vi "Parameter.vi"(9 "In":string, 10 "VIId":string, 11 "VariablesRef":T3) -> ()   [LabVIEW 2018, in "File.lvlib"]
uses:
  File.lvlib
  <userlib>/_OpenG.lib/dictionary/dictionary.llb/Dictionary Object RefNum__ogtk.ctl
  <userlib>/_OpenG.lib/dictionary/dictionary.llb/Dictionary Object RefNum - Enum__ogtk.ctl
  <vilib>/addons/_JKI.lib/Serialization/JSON/JKI JSON Serialization.lvlib
panel:
  in  "Tab Control":enum32{"Config", "控件"}(tab)
  in  "Type":T1(tab)
  in  "路径类型_SetPath":u16(ring) items=["Relative", "Absolute"]
  in  "禁用缓存_CreatFile":bool
  in  "权限_CreatFile":u16(ring) caption="权限" items=["read/write", "read-only", "write-only"]
  in  "操作_CreatFile":u16(ring) caption="操作" items=["open", "replace", "create", "open or create", "replace or create", "replace or create with confirmation"]
  in  "手动确认_Delete":bool
  in  "完整层次结构_Delete":bool
  in  "计数_ReadTextFile":i32=-1 caption="计数"
  in  "文本_WriteTextFile":string(combo) caption="文本"
  in  "起始位置_WriteTextFile":u16(ring) caption="起始位置" items=["start", "end", "current"]
  in  "偏移_WriteTextFile":i64 caption="偏移"
  in  "计数_ReadBinFile":i32=-1 caption="计数"
  in  "字节顺序_ReadBinFile":u16(ring) caption="字节顺序" items=["big-endian, network order", "native, host order", "little-endian"]
  in  "前置数据大小_WriteBinFile":bool=TRUE
  in  "字节顺序_WriteBinFile":u16(ring) items=["big-endian, network order", "native, host order", "little-endian"]
  in  "二进制_WriteBinFile":string(combo) caption="二进制内容"
  in  "覆盖_Move":bool
  in  "文件路径_Move":string(combo) caption="目标文件路径"
  in  "目标文件路径_Copy":string(combo) caption="目标文件路径"
  in  "覆盖_Copy":bool
  in  "类型_ListFolder":u16(ring) caption="类型" items=["File", "Folder"]
  in  "方法(Method)":T2(ring)
  in  "路径(Path)":string(combo)
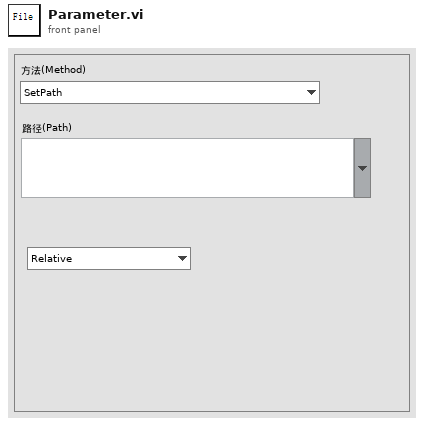
[diagram p1: front panel]
types:
  T1 = enum32{"SetPath", "CreatFile", "CreatFolder", "Delete", "ReadTextFile", "WriteTextFile", "ReadBinFile", "WriteBinFile", "ReadFileMD5", "Move", "Copy", "GetFileSize", "CheckifFileorFolderExists", "ListFolder"}
  T2 = enum16{"SetPath", "CreatFile", "CreatFolder", "Delete", "ReadTextFile", "WriteTextFile", "ReadBinFile", "WriteBinFile", "ReadFileMD5", "Move", "Copy", "GetFileSize", "CheckifFileorFolderExists", "ListFolder"}
  T3 = typedef "Dictionary Object RefNum__ogtk.ctl" = refnum<k1>
  T4 = cluster{"SetPath":cluster{"json":cluster{"Method":string, "Path":string, "PathType":string}}, "CreatFile":cluster{"json":cluster{"Method":string, "Path":string, "Operation":string, "Access":string, "DisableBuffering":bool}}, "CreatFolder":cluster{"json":cluster{"Method":string, "Path":string}}, "Delete":cluster{"json":cluster{"Method":string, "Path":string, "EntireHierarchy":bool, "Confirm":bool}}, "ReadTextFile":cluster{"json":cluster{"Method":string, "Path":string, "count":i32}}, "WriteTextFile":cluster{"json":cluster{"Method":string, "Path":string, "Offset":i64, "Position":string, "Text":string}}, "ReadBinFile":cluster{"json":cluster{"Method":string, "Path":string, "Count":i32, "ByteOrder":string}}, "WriteBinFile":cluster{"json":cluster{"Method":string, "Path":string, "ByteOrder":string, "PrependDataSize":bool, "Bin":string}}, "ReadFileMD5":cluster{"json":cluster{"Method":string, "Path":string}}, "Move":cluster{"json":cluster{"Method":string, "Path":string, "TargetPath":string, "Overwrite":bool}}, "Copy":cluster{"json":cluster{"Method":string, "Path":string, "TargetPath":string, "Overwrite":bool}}, "GetFileSize":cluster{"json":cluster{"Method":string, "Path":string}}, "CheckifFileorFolderExists":cluster{"json":cluster{"Method":string, "Path":string}}, "ListFolder":cluster{"json":cluster{"Method":string, "Path":string, "Type":string}}}
  T5 = enum32{"Invalid", "Standard", "Closed", "Hidden", "Minimized", "Maximized"}
  T6 = enum32{"invalid app kind", "Development System", "Run Time System", "Student Edition", "Embedded LabVIEW", "Evaluation", "Custom"}
  T7 = cluster{"Core":cluster{"Current VI Reference":refnum<vi>, "Close Panel on Exit?":bool}, "Parameter":cluster{"VariableRef":T3}, "Synchronize":cluster{"EnqueueData":cluster{"Action":enum16{"Create", "Query", "Revert", "UpdateVariable", "Close"}, "Data":variant}, "Echo":cluster{"VIRef":refnum<vi>, "JsonOut":string, "Status":string}, "Communicate":cluster{"ID":string, "JsonIn":string, "VarRef":T3}, "Queue":refnum<queue>}, "FileClusters":cluster{"SetPath":cluster{"json":cluster{"Method":string, "Path":string, "PathType":string}}, "CreatFile":cluster{"json":cluster{"Method":string, "Path":string, "Operation":string, "Access":string, "DisableBuffering":bool}}, "CreatFolder":cluster{"json":cluster{"Method":string, "Path":string}}, "Delete":cluster{"json":cluster{"Method":string, "Path":string, "EntireHierarchy":bool, "Confirm":bool}}, "ReadTextFile":cluster{"json":cluster{"Method":string, "Path":string, "count":i32}}, "WriteTextFile":cluster{"json":cluster{"Method":string, "Path":string, "Offset":i64, "Position":string, "Text":string}}, "ReadBinFile":cluster{"json":cluster{"Method":string, "Path":string, "Count":i32, "ByteOrder":string}}, "WriteBinFile":cluster{"json":cluster{"Method":string, "Path":string, "ByteOrder":string, "PrependDataSize":bool, "Bin":string}}, "ReadFileMD5":cluster{"json":cluster{"Method":string, "Path":string}}, "Move":cluster{"json":cluster{"Method":string, "Path":string, "TargetPath":string, "Overwrite":bool}}, "Copy":cluster{"json":cluster{"Method":string, "Path":string, "TargetPath":string, "Overwrite":bool}}, "GetFileSize":cluster{"json":cluster{"Method":string, "Path":string}}, "CheckifFileorFolderExists":cluster{"json":cluster{"Method":string, "Path":string}}, "ListFolder":cluster{"json":cluster{"Method":string, "Path":string, "Type":string}}}}
  T8 = cluster{"EnqueueData":cluster{"Action":enum16{"Create", "Query", "Revert", "UpdateVariable", "Close"}, "Data":variant}, "Echo":cluster{"VIRef":refnum<vi>, "JsonOut":string, "Status":string}, "Communicate":cluster{"ID":string, "JsonIn":string, "VarRef":T3}, "Queue":refnum<queue>}
  T9 = cluster{"Current VI Reference":refnum<vi>, "Close Panel on Exit?":bool}
  T10 = cluster{"json":cluster{"Method":string, "Path":string, "PathType":string}}
  T11 = cluster{"json":cluster{"Method":string, "Path":string, "Operation":string, "Access":string, "DisableBuffering":bool}}
  T12 = cluster{"json":cluster{"Method":string, "Path":string}}
  T13 = cluster{"json":cluster{"Method":string, "Path":string, "EntireHierarchy":bool, "Confirm":bool}}
  T14 = cluster{"json":cluster{"Method":string, "Path":string, "count":i32}}
  T15 = cluster{"json":cluster{"Method":string, "Path":string, "Offset":i64, "Position":string, "Text":string}}
  T16 = cluster{"json":cluster{"Method":string, "Path":string, "Count":i32, "ByteOrder":string}}
  T17 = cluster{"json":cluster{"Method":string, "Path":string, "ByteOrder":string, "PrependDataSize":bool, "Bin":string}}
  T18 = cluster{"json":cluster{"Method":string, "Path":string, "TargetPath":string, "Overwrite":bool}}
  T19 = cluster{"json":cluster{"Method":string, "Path":string, "Type":string}}
  T20 = cluster{"Action":enum16{"Create", "Query", "Revert", "UpdateVariable", "Close"}, "Data":variant}
  T21 = cluster{"ID":string, "JsonIn":string, "VarRef":T3}
  T22 = enum16{"Create", "Query", "Revert", "UpdateVariable", "Close"}
  T23 = cluster{"VIRef":refnum<vi>, "JsonOut":string, "Status":string}
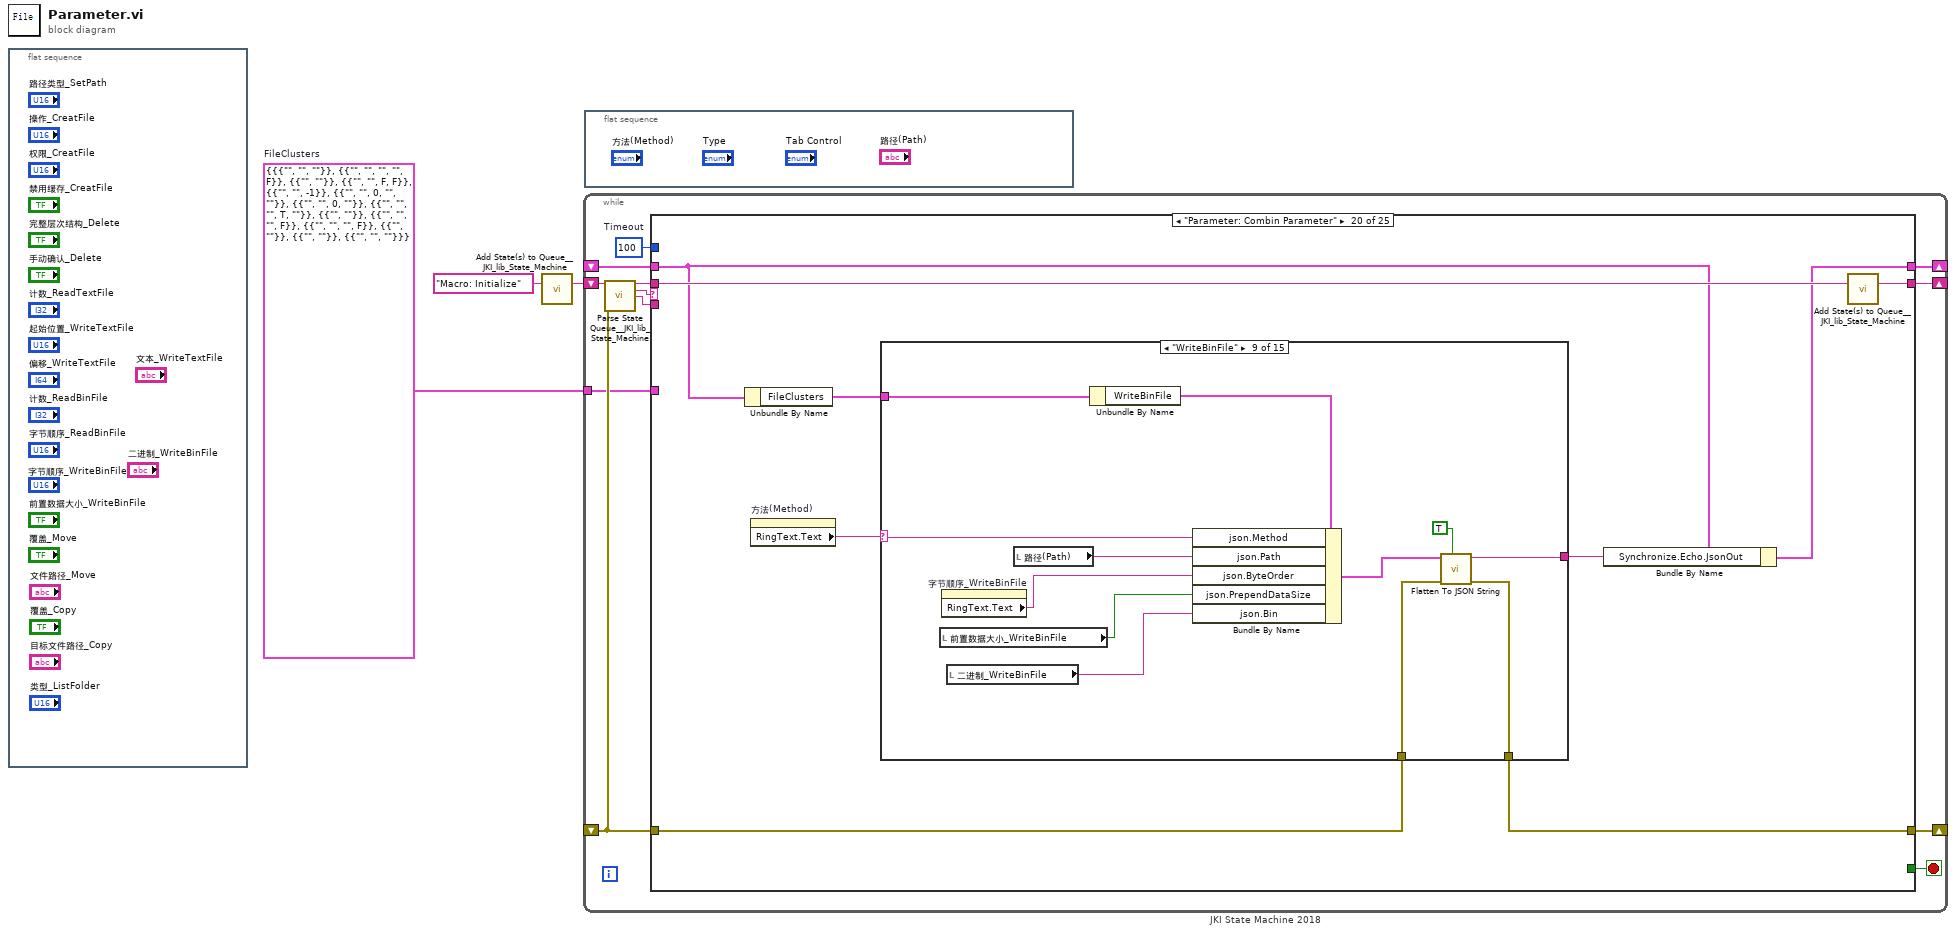
[diagram p0: block diagram]
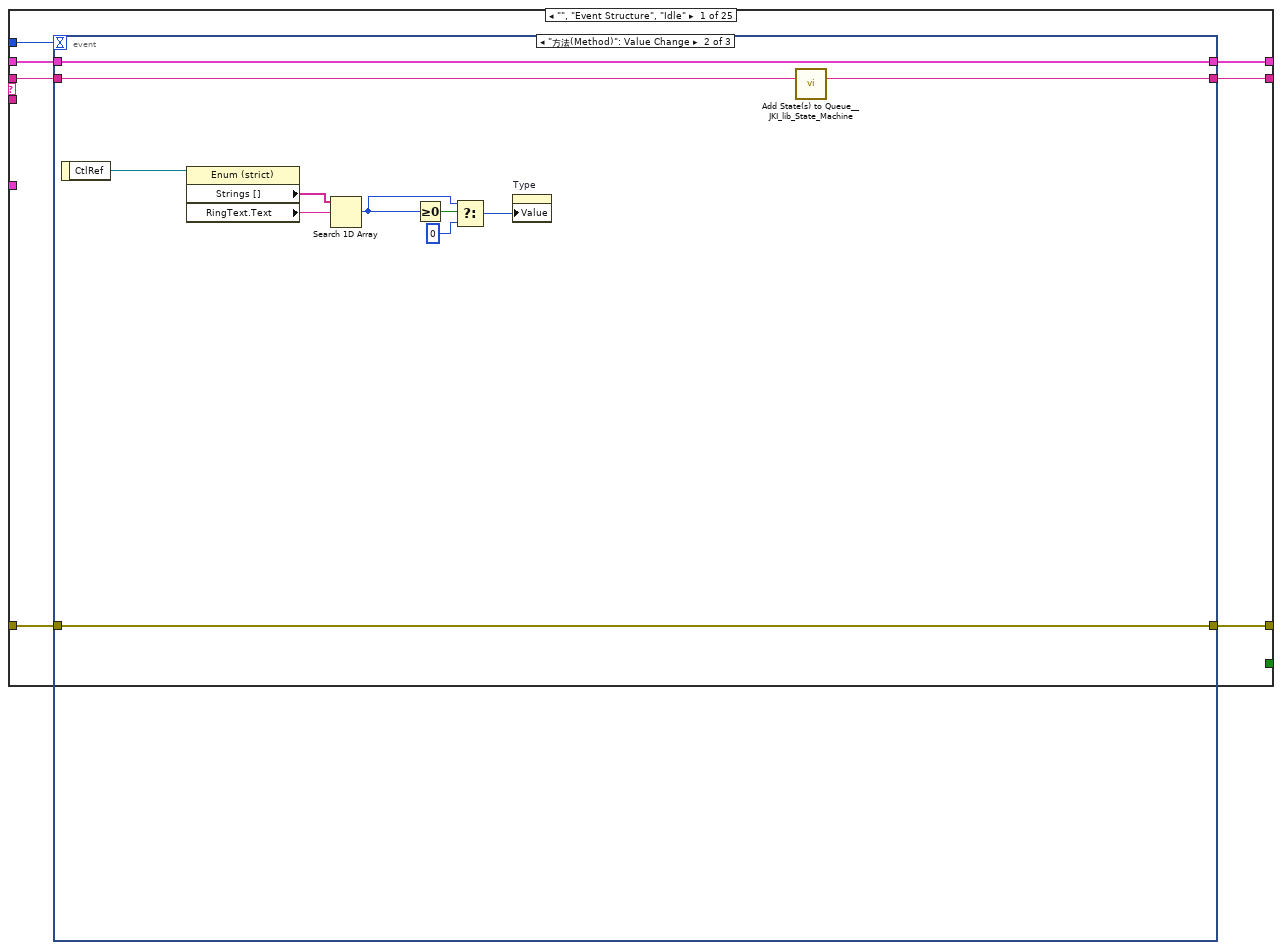
[diagram p2: hidden frame]
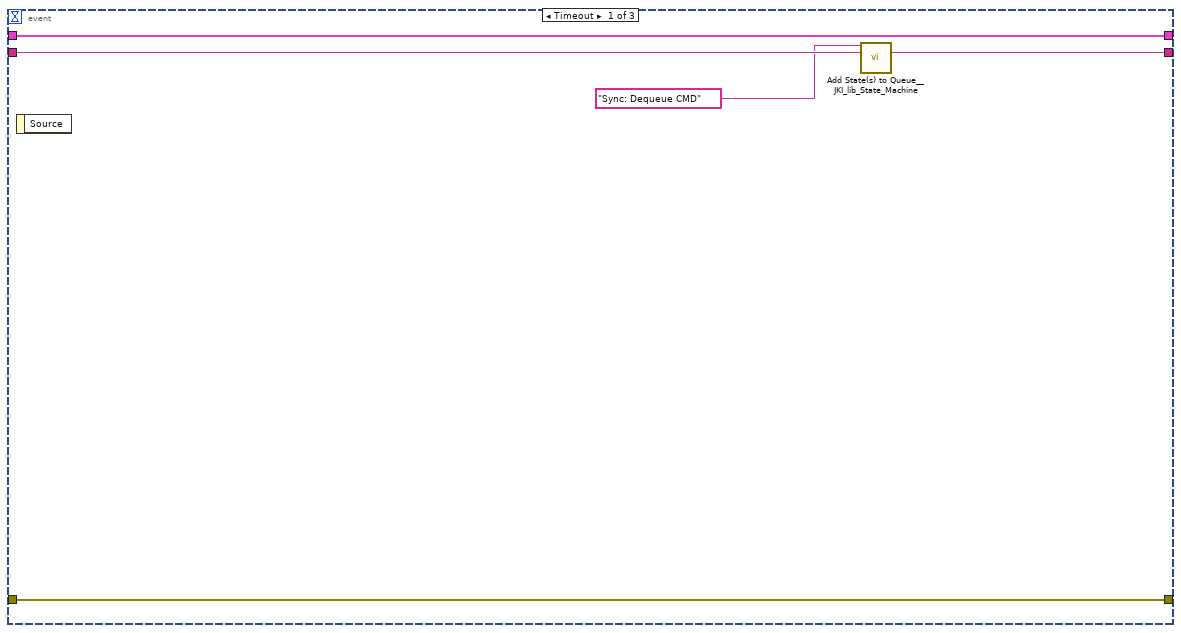
[diagram p3: hidden frame]
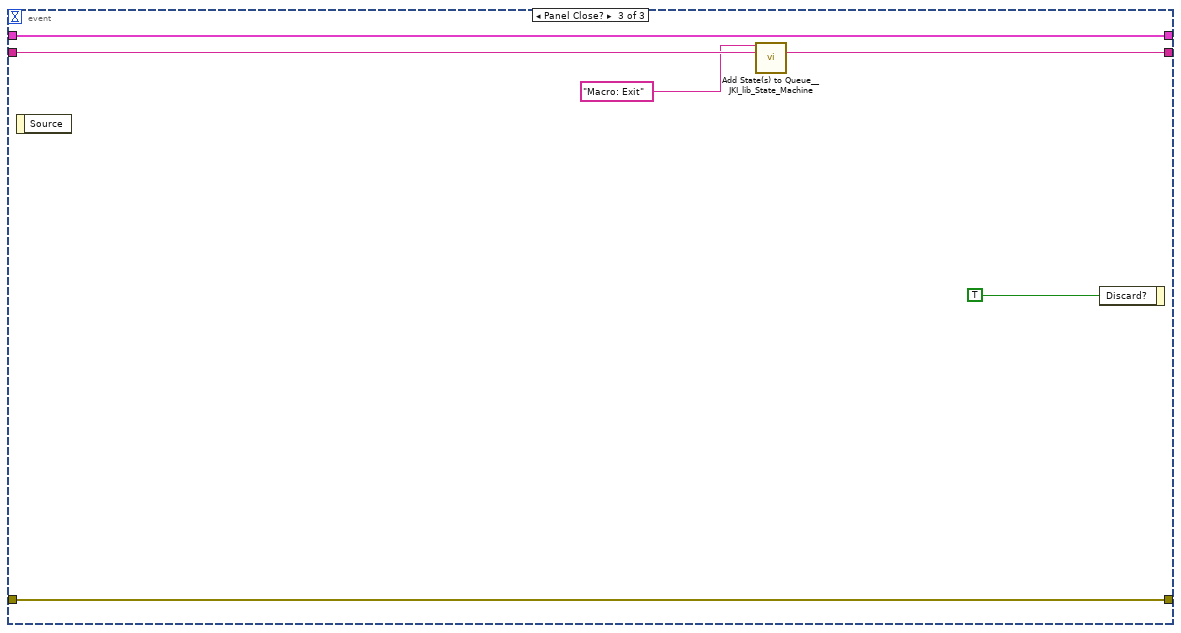
[diagram p4: hidden frame]
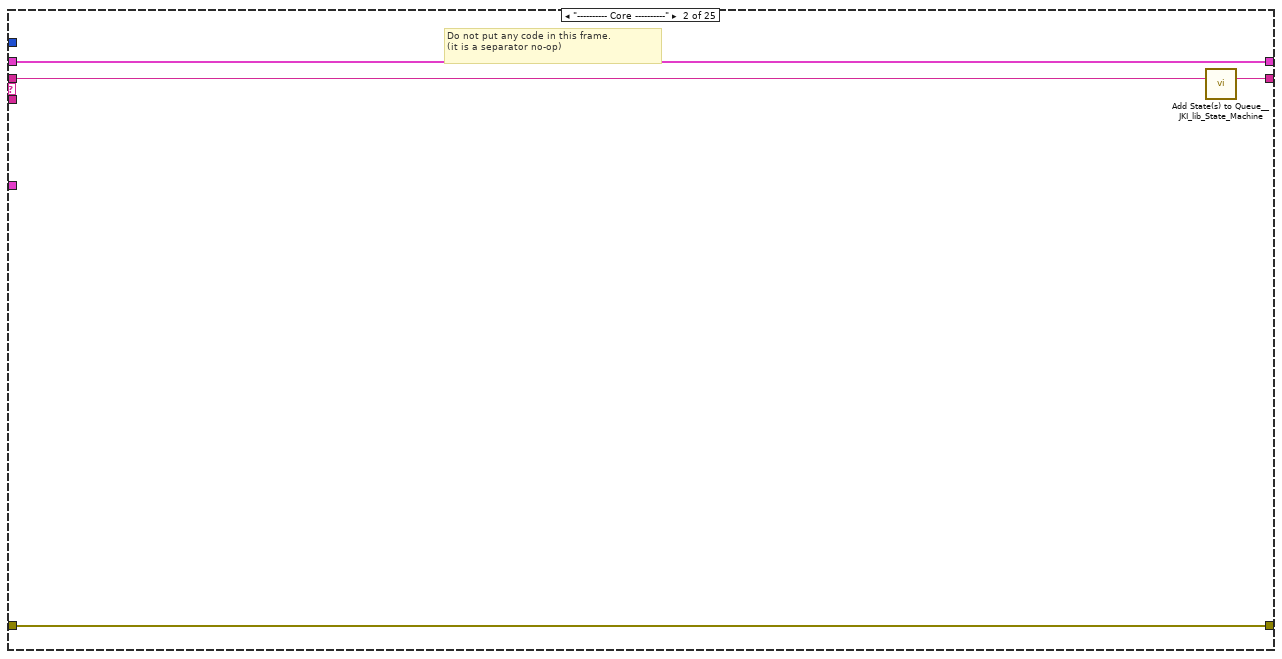
[diagram p5: hidden frame]
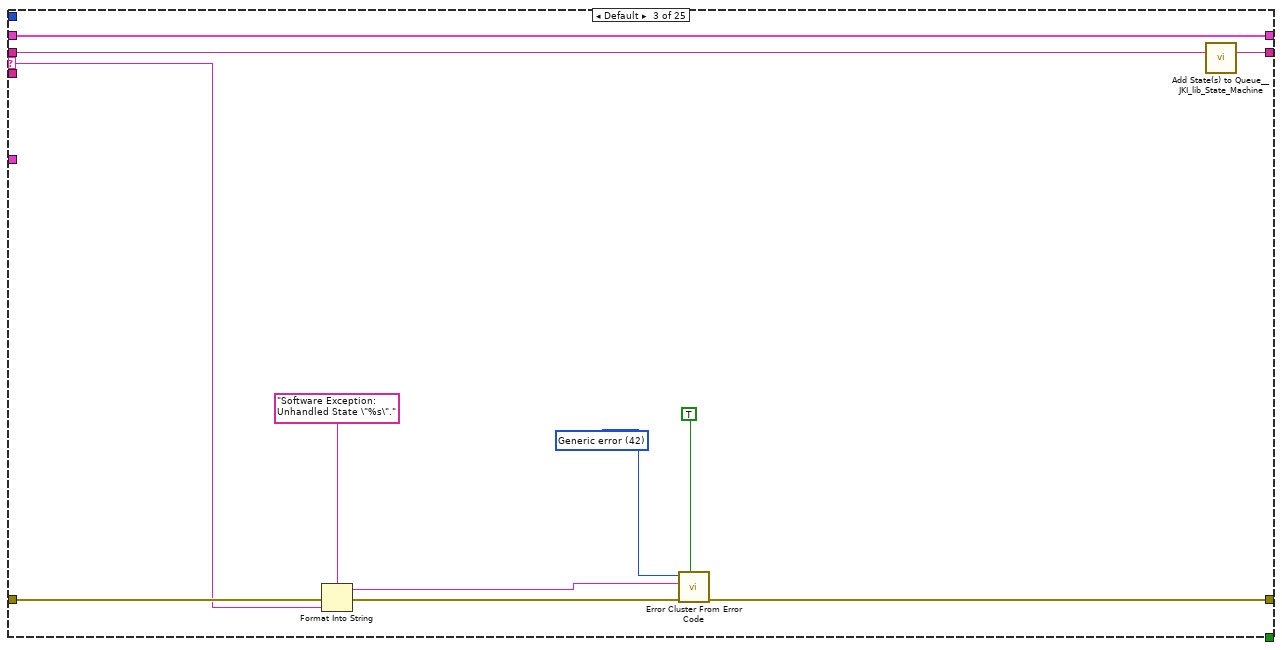
[diagram p6: hidden frame]
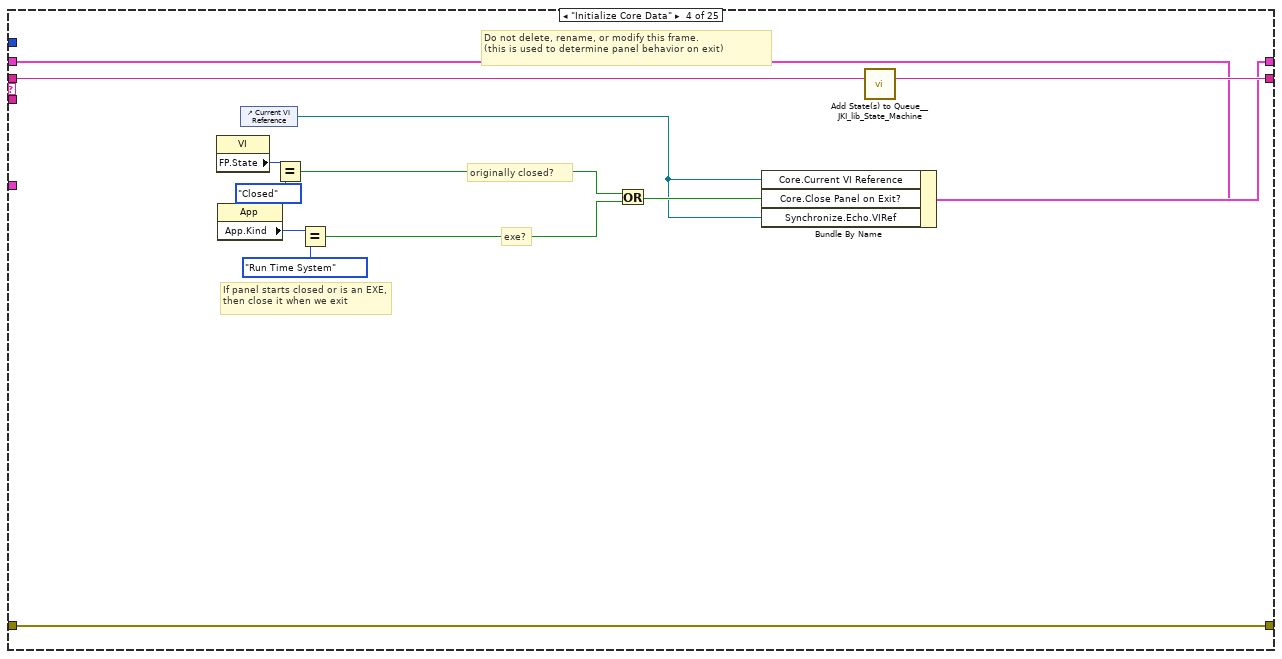
[diagram p7: hidden frame]
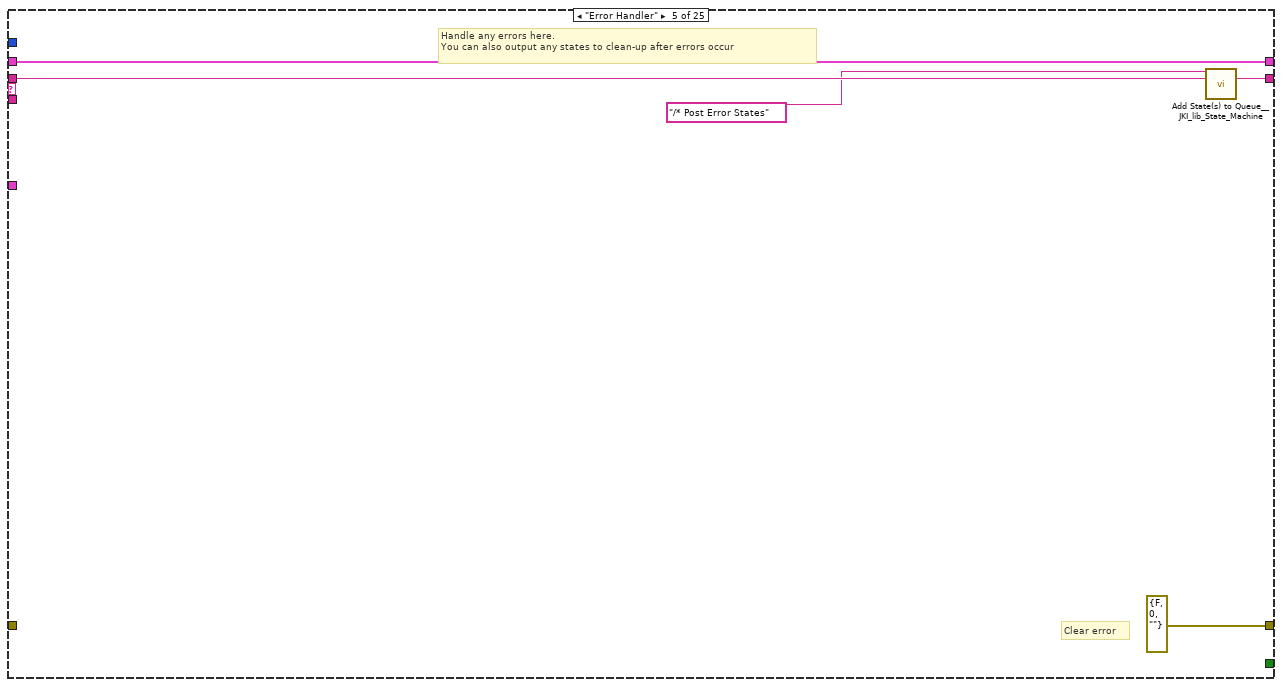
[diagram p8: hidden frame]
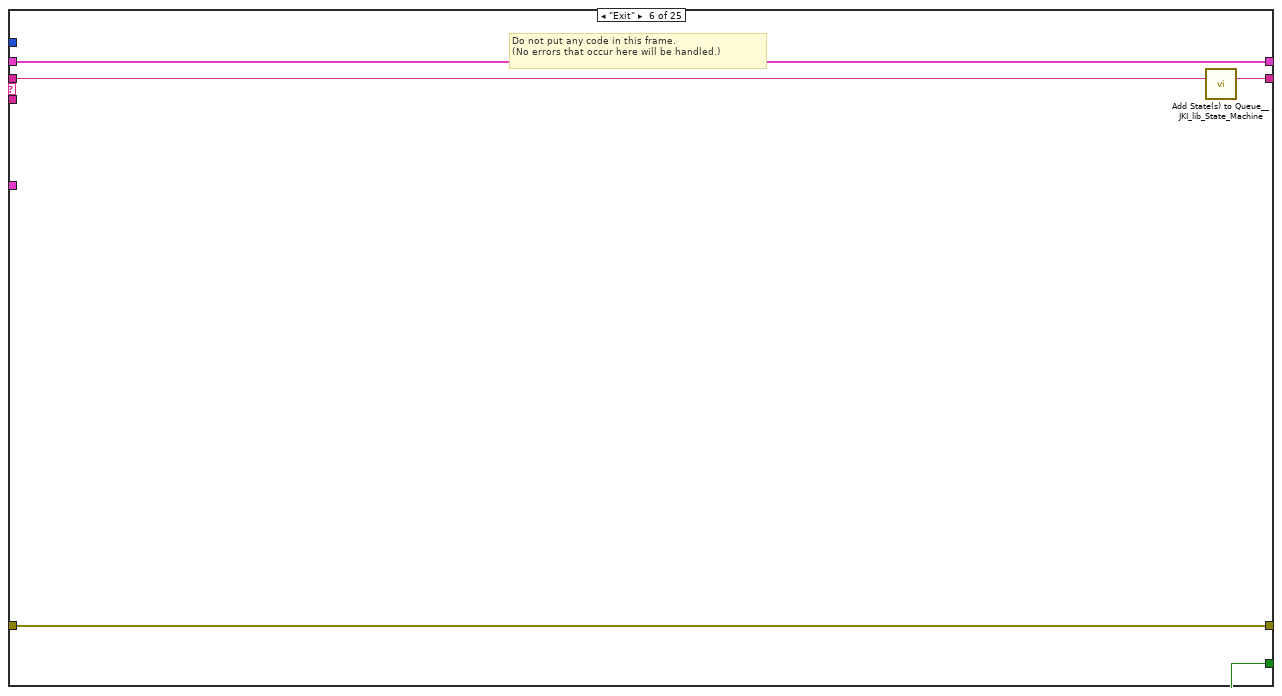
[diagram p9: hidden frame]
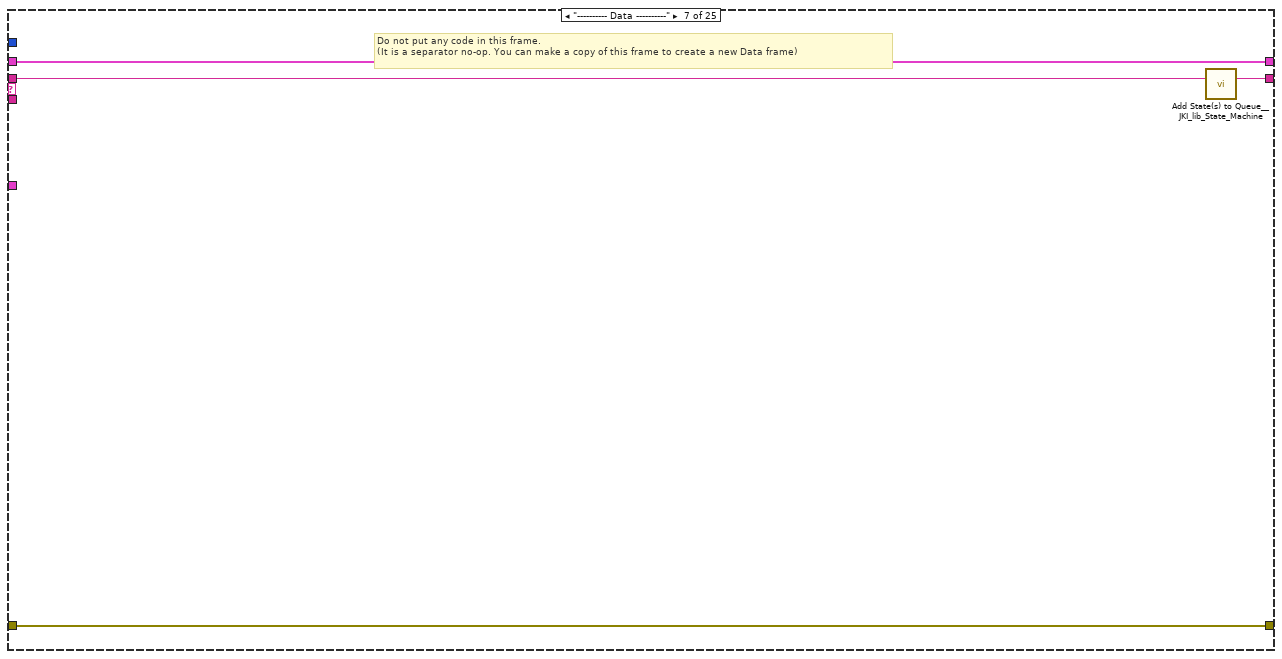
[diagram p10: hidden frame]
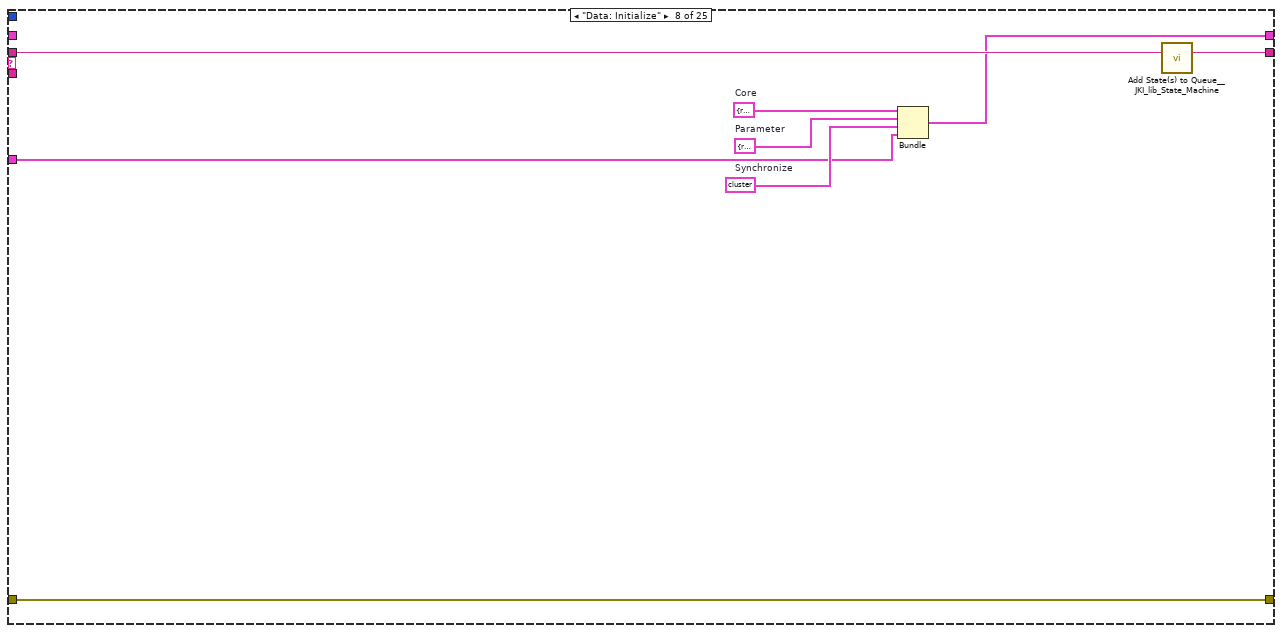
[diagram p11: hidden frame]
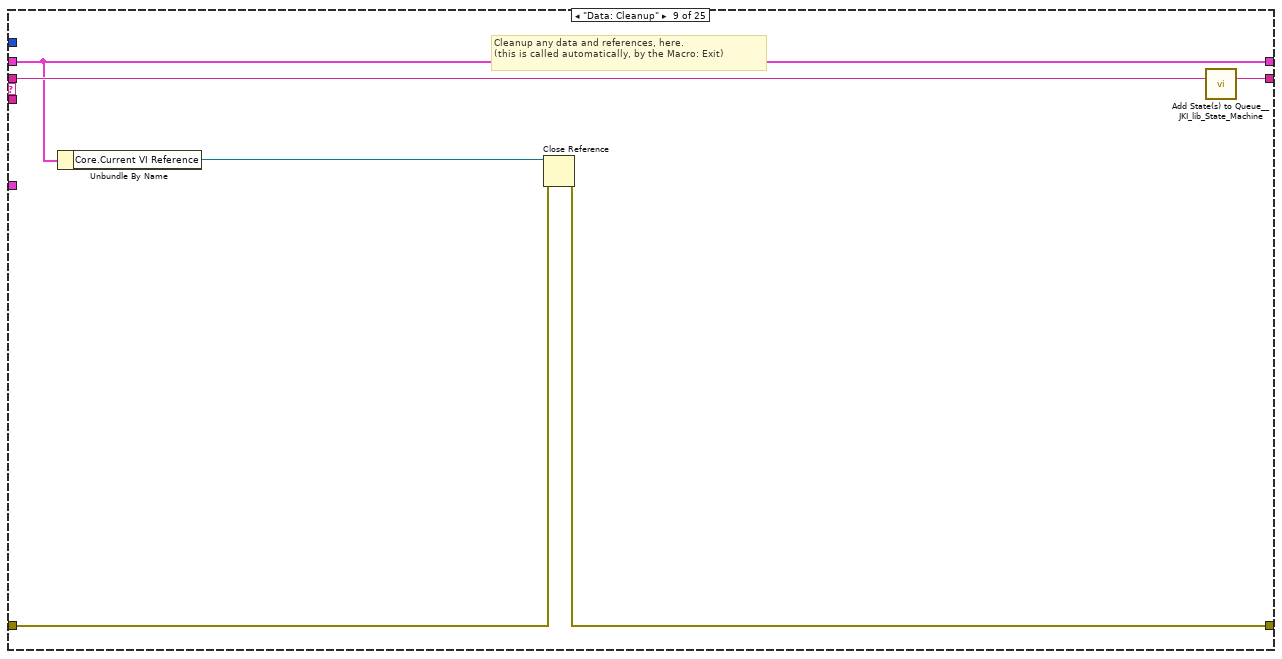
[diagram p12: hidden frame]
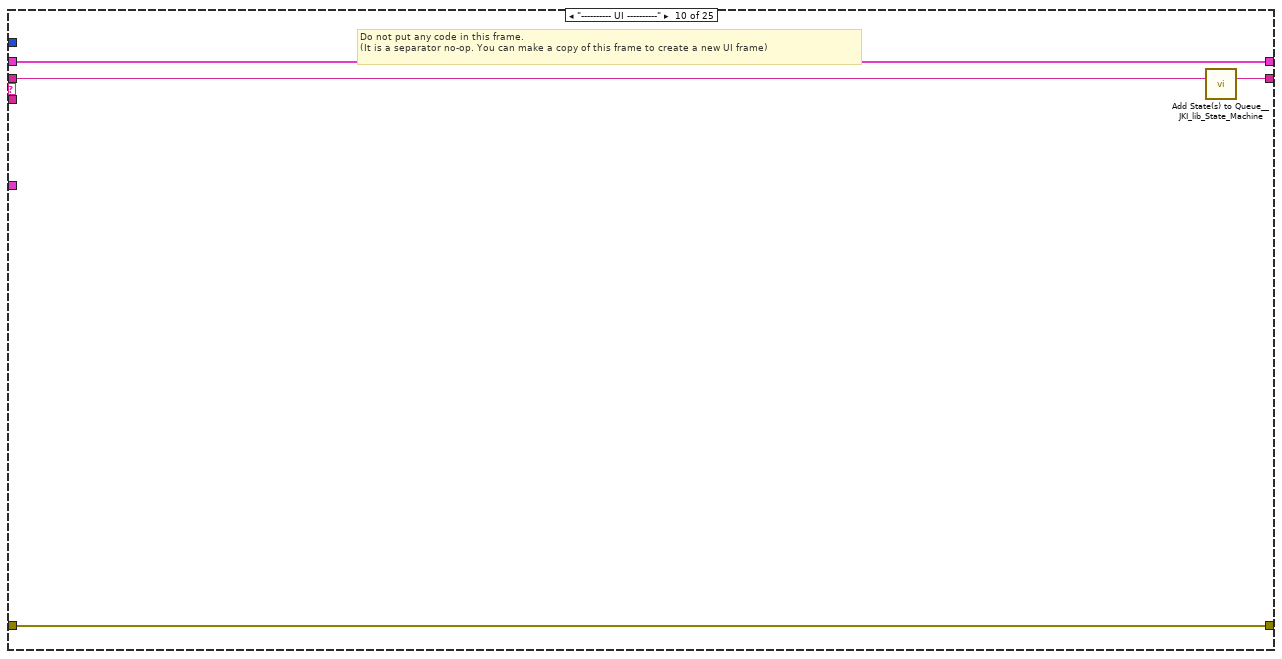
[diagram p13: hidden frame]
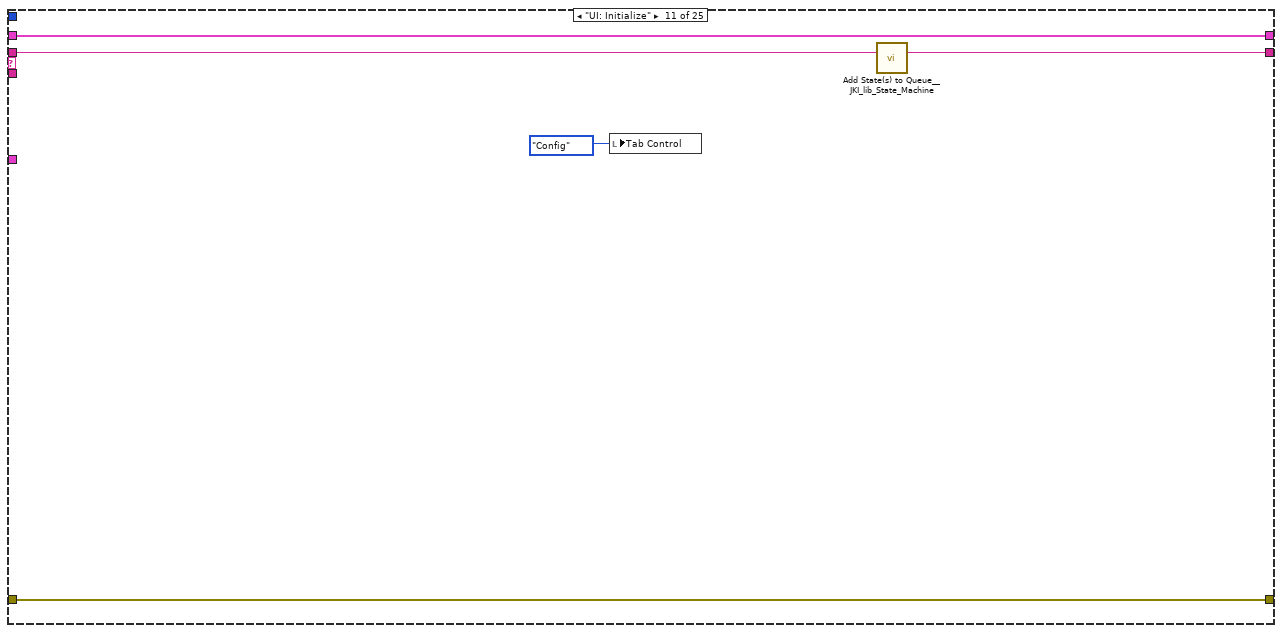
[diagram p14: hidden frame]
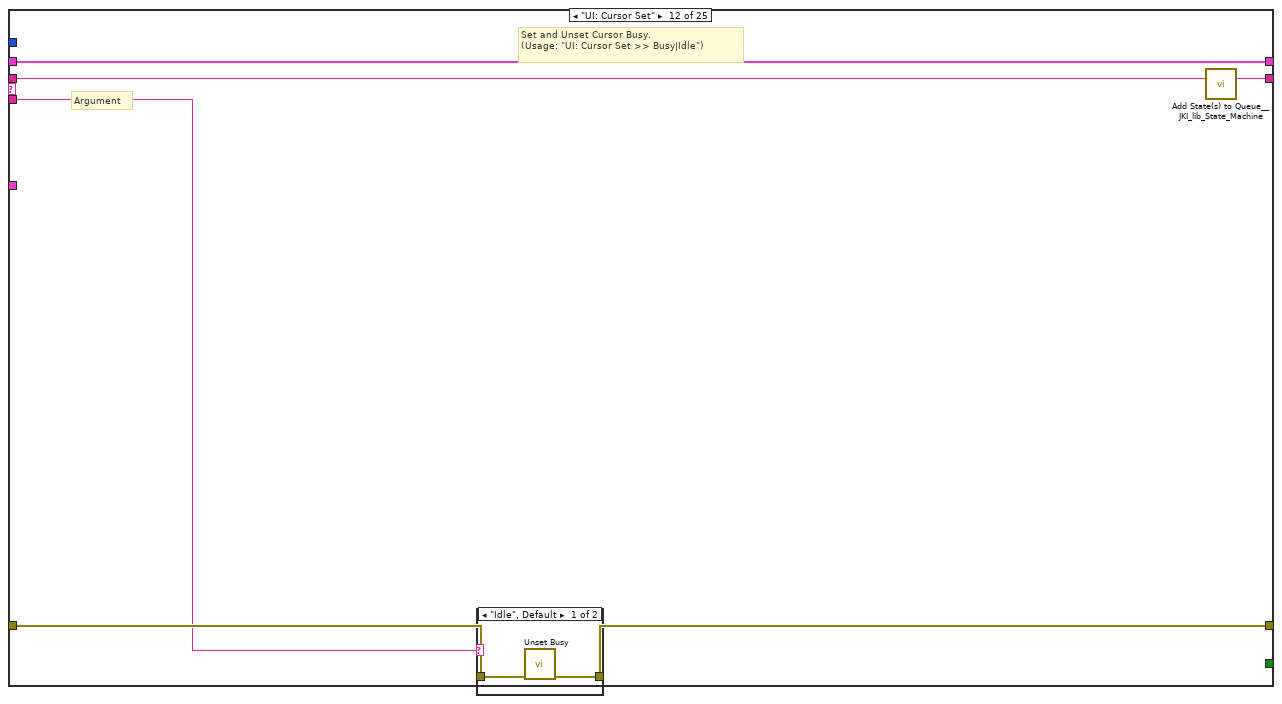
[diagram p15: hidden frame]
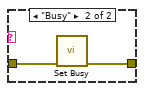
[diagram p16: hidden frame]
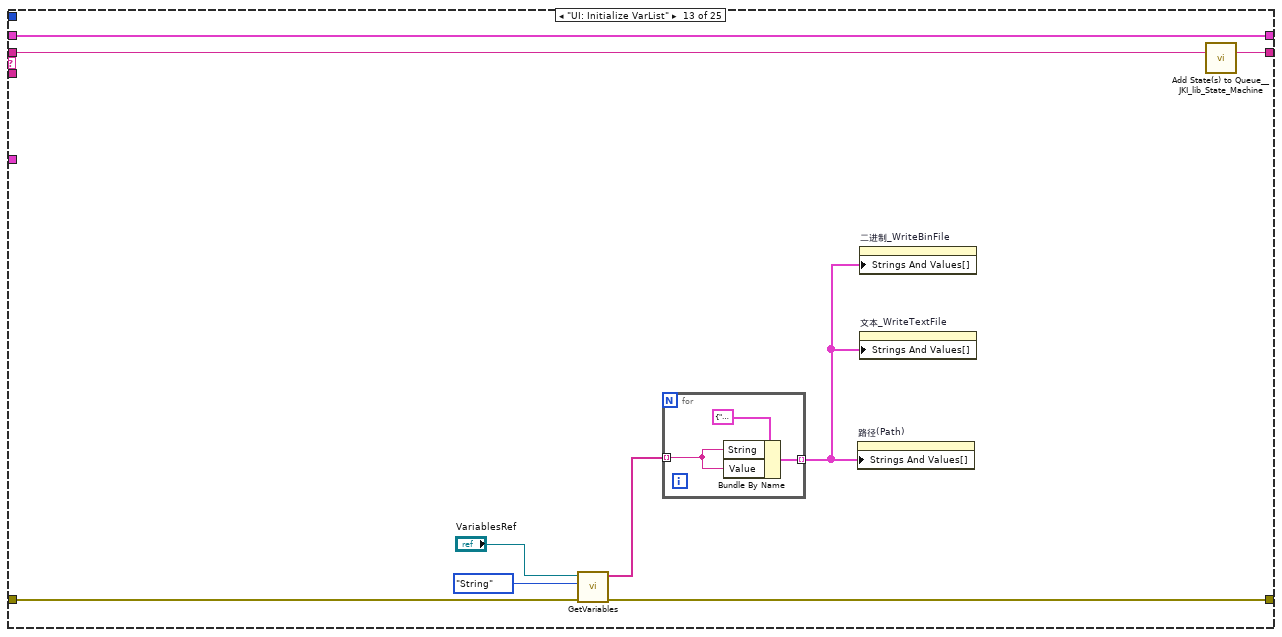
[diagram p17: hidden frame]
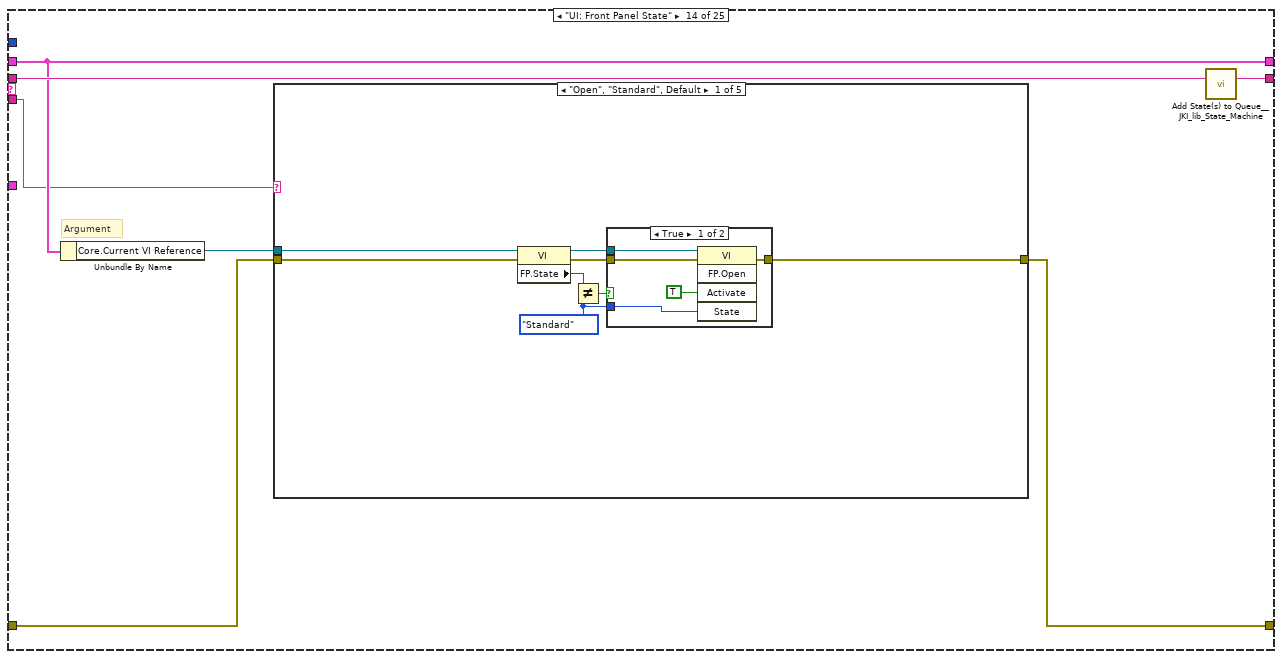
[diagram p18: hidden frame]
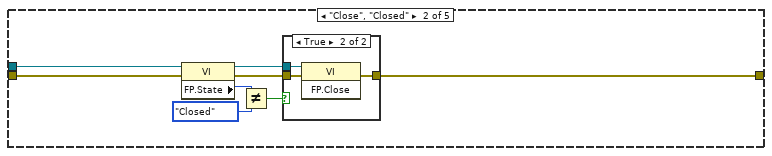
[diagram p20: hidden frame]
diagram:
  w1 = T4 {"SetPath"={"json"={"Method"="", "Path"="", "PathType"=""}}, "CreatFile"={"json"={"Method"="", "Path"="", "Operation"="", "Access"="", "DisableBuffering"=FALSE}}, "CreatFolder"={"json"={"Method"="", "Path"=""}}, "Delete"={"json"={"Method"="", "Path"="", "EntireHierarchy"=FALSE, "Confirm"=FALSE}}, "ReadTextFile"={"json"={"Method"="", "Path"="", "count"=-1}}, "WriteTextFile"={"json"={"Method"="", "Path"="", "Offset"=0, "Position"="", "Text"=""}}, "ReadBinFile"={"json"={"Method"="", "Path"="", "Count"=0, "ByteOrder"=""}}, "WriteBinFile"={"json"={"Method"="", "Path"="", "ByteOrder"="", "PrependDataSize"=TRUE, "Bin"=""}}, "ReadFileMD5"={"json"={"Method"="", "Path"=""}}, "Move"={"json"={"Method"="", "Path"="", "TargetPath"="", "Overwrite"=FALSE}}, "Copy"={"json"={"Method"="", "Path"="", "TargetPath"="", "Overwrite"=FALSE}}, "GetFileSize"={"json"={"Method"="", "Path"=""}}, "CheckifFileorFolderExists"={"json"={"Method"="", "Path"=""}}, "ListFolder"={"json"={"Method"="", "Path"="", "Type"=""}}}  # FileClusters
  n1 = flat-sequence {
    frame #0 {
    }
  }
  n2 = call <vilib>:"Add State(s) to Queue__JKI_lib_State_Machine.vi"("State(s) in (\"\")"="Macro: Initialize") -> ("States Out"=w3:string)  [unwired: 14 in]
  n3 = while "JKI State Machine 2018" {
    shift-right: [w8] -> _
    shift-left: _ -> [w7]
    shift-right: [w11] -> _
    shift-left: _ -> [w5]
    shift-right: [w10] -> _
    shift-left: w3 -> [w12]
    tunnel: w1 -> [w4]
    stop <- w9 stop-if-true
    w6 = 100  # Timeout
    n4 = call <vilib>:"Parse State Queue__JKI_lib_State_Machine.vi"("State Queue"=w12, "Error In (no error)"=w5) -> ("Remaining States"=w14:string, "Current State"=w15:string, "Arguments"=w13:string)  [unwired: 11 in]
    n5 = case shown="\"Parameter: Combin Parameter\"" w15 {
      selector: w15 -> [_ _ w49 _ _ _ _ _ _ _ _ _ _ _ _ _ _ _ _ _ _ _ _ _ _]
      tunnel: w14 -> [w22 w48 w53 w72 w77 w82 w86 w94 w100 w104 w109 w115 w128 w138 w207 w212 w222 w226 w234 w454 w605 w614 w629 w673 w688]
      tunnel: w13 -> [_ _ _ _ _ _ _ _ _ _ _ w110 _ w132 _ _ _ _ _ _ _ _ _ _ _]
      tunnel: w7 -> [w20 w45 w51 w65 w74 w80 w83 _ w95 w101 w106 w113 w126 w134 w204 w209 w219 w223 w229 w447 w602 w607 w627 w670 w677]
      tunnel: [w19 w46 w55 w69 errorcluster {"status"=FALSE, "code"=0, "source"=""} ("error out") w79 w84 w92 w96 w102 w105 w111 w122 w135 w205 w210 w220 w224 w230 w451 w603 w611 w616 w668 w675] -> w11
      tunnel: w5 -> [w18 w46 w54 w69 _ w79 w84 w92 w97 w102 w105 w112 w123 w136 w205 w210 w220 w224 w231 w450 w603 w612 w625 w669 w676]
      tunnel: [w21 w47 w52 w71 w76 w81 w85 w93 w99 w103 w108 w114 w127 w137 w206 w211 w221 w225 w233 w453 w604 w613 w628 w672 w687] -> w10
      tunnel: [_ _ _ _ _ TRUE _ _ _ _ _ _ _ _ _ _ _ _ _ _ _ _ _ _ _] -> w9
      tunnel: [w17 w45 w51 w70 w74 w80 w83 w89 w95 w101 w106 w113 w126 w134 w204 w209 w219 w223 w229 w452 w602 w609 w618 w670 w677] -> w8
      tunnel: w6 -> [w16 _ _ _ _ _ _ _ _ _ _ _ _ _ _ _ _ _ _ _ _ _ _ _ _]
      tunnel: w4 -> [_ _ _ _ _ _ _ w87 _ _ _ _ _ _ _ _ _ _ _ _ _ _ _ _ _]
      frame "", "Event Structure", "Idle" {
        n6 = event shown="[1] \"方法(Method)\": Value Change" {
          selector: _ -> [_ _ _]
          dyn-events: _ -> [_ _ _]
          timeout: w16 -> [_ _ _]
          tunnel: w22 -> [w27 w38 w44]
          tunnel: [w26 w37 w43] -> w21
          tunnel: w20 -> [w24 w35 w41]
          tunnel: [w25 w36 w42] -> w19
          tunnel: w18 -> [w25 w36 w42]
          tunnel: [w24 w35 w41] -> w17
          event Timeout {
            n7 = event-data() -> ()  [unwired: 1 in, 1 out]
            n8 = call <vilib>:"Add State(s) to Queue__JKI_lib_State_Machine.vi"("State(s) in Front (\"\")"="Sync: Dequeue CMD" ("State(s) in Front (\"\")"), "State(s) in (\"\")"=w27) -> ("States Out"=w26:string)  [unwired: 13 in]
          }
          event "方法(Method)": Value Change {
            n9 = event-data() -> ("CtlRef"=w31:refnum<vi>)  [unwired: 1 in]
            n10 = property class="Enum (strict)"(reference=w31) -> ("Strings []"=w30:string[], "RingText.Text"=w29:string)  [unwired: 1 in, 2 out]
            n11 = Search 1D Array(1D array=w30, element=w29) -> (index of element=w33:i32)  [unwired: 1 in]
            n12 = Greater Or Equal To 0?(x=w33) -> (x >= 0?=w34:bool)
            n13 = Select(t=w33, s=w34, f=0) -> (s? t:f=w28:i32)
            n14 = property on="Type" class="TabCtl (strict)"("Value"=w28) -> ()  [unwired: 2 in, 2 out]
            n15 = call <vilib>:"Add State(s) to Queue__JKI_lib_State_Machine.vi"("State(s) in (\"\")"=w38) -> ("States Out"=w37:string)  [unwired: 14 in]
          }
          event Panel Close? {
            n16 = event-data() -> ()  [unwired: 1 in, 1 out]
            n17 = call <vilib>:"Add State(s) to Queue__JKI_lib_State_Machine.vi"("State(s) in Front (\"\")"="Macro: Exit", "State(s) in (\"\")"=w44) -> ("States Out"=w43:string)  [unwired: 13 in]
            n18 = event-data("Discard?"=TRUE) -> ()  [unwired: 1 in, 1 out]
          }
        }
      }
      frame "---------- Core ----------" {
        # "Do not put any code in this frame.\n(it is a separator no-op)"
        n19 = call <vilib>:"Add State(s) to Queue__JKI_lib_State_Machine.vi"("State(s) in (\"\")"=w48) -> ("States Out"=w47:string)  [unwired: 14 in]
      }
      frame Default {
        w58 = 42 items=["No error", "Argument error", "Memory is full", "Out of zone", "End of file", "File already open", "Generic file I/O error", "File not found", "File permission error", "Disk is full", "Duplicate path", "Too many files open", "System feature not enabled", "Resource file not found", "Cannot add resource", "Resource not found", "Image not found", "Image memory error", "Pen does not exist", "Config type invalid", "Config token not found", "Config parse error", "Config memory error", "Bad external code format", "Bad external code offset", "External code not present", "Null window", "Destroy window error", "Null menu", "Print aborted", "Bad print record", "Print driver error", "Windows error during printing", "Memory error during printing", "Print dialog error", "Generic print error", "Invalid device refnum", "Device not found", "Device parameter error", "Device unit error", "Cannot open device", "Device call aborted", "Generic error", "Cancelled by user", "Object ID too low", "Object ID too high", "Object not in heap", "Unknown heap", "Unknown object (invalid DefProc)", "Unknown object (DefProc not in table)", "Message out of range", "Invalid (null) method", "Unknown message", "Manager call not supported", "Bad address", "Network operation in progress", "Network operation timed out", "Connection is busy", "Network attribute not supported", "Network error", "Address in use", "System out of memory", "Connection aborted", "Connection refused", "Not connected", "Already connected", "Connection closed", "Initialization error (interapplication manager)", "Bad occurrence", "Wait on unbound occurrence handler", "Occurrence queue overflow", "Datalog type conflict", "Unused", "Unrecognized type (interapplication manager)", "Memory corrupt", "Failed to make temporary DLL", "Old CIN version", "Drag socket not found", "Failed to load drop-object", "Failed to register OLE object", "Failed to release OLE object", "Format specifier type mismatch", "Unknown format specifier", "Too few format specifiers", "Too many format specifiers", "Scan failed", "Newer CIN version", "Error converting to variant", "Runtime menu error", "Password tampered", "Variant attribute not found", "Incompatible variant data type", "Event data is not available", "Event Store is not present", "Occurrence is not found", "Event Queue is not created", "Event info is not available", "Refnum passed is NULL", "Error retrieving Class GUID", "Error retrieving CoClass GUID", "Error retrieving TypeLib GUID.", "Bad built application magic bytes.", "Specific driver is different from the specific driver associated with the Logical Name.", "There is no session opened to the class driver.", "Max Error", "MAX - Error with config objects", "MAX - Error loading configuration", "MAX - Group not supported"]
        n20 = Format Into String(format string="Software Exception: Unhandled State \"%s\"." ("message"), error in=w54, w49) -> (resulting string=w57:string, error out=w56:errorcluster)  [unwired: 1 in]
        n21 = call <vilib>:"Error Cluster From Error Code.vi"("show call chain? (False)"=TRUE, "error in (no error)"=w56, "error message (\"\")"=w57, "error code (0)"=w58) -> ("error out"=w55:errorcluster)  [unwired: 5 in]
        n22 = call <vilib>:"Add State(s) to Queue__JKI_lib_State_Machine.vi"("State(s) in (\"\")"=w53) -> ("States Out"=w52:string)  [unwired: 14 in]
      }
      frame "Initialize Core Data" {
        # "Do not delete, rename, or modify this frame.\n(this is used to determine panel behavior on exit)"
        # "originally closed?"
        # "exe?"
        # "If panel starts closed or is an EXE, then close it when we exit"
        n23 = property class="VI"() -> ("FP.State"=w63:T5)  [unwired: 2 in, 2 out]
        n24 = property class="App"() -> ("App.Kind"=w68:T6)  [unwired: 2 in, 2 out]
        n25 = control-ref of="Current VI Reference"() -> (w60:refnum<vi>)
        n26 = Equal?(x=w63, y=T5."Closed" ("Front Panel Window:State")) -> (x = y?=w61:bool)
        n27 = Equal?(x=w68, y=T6."Run Time System" ("Application:Kind")) -> (x = y?=w66:bool)
        n28 = Or(x=w61, y=w66) -> (x .or. y?=w64:bool)
        n29 = Bundle By Name(cluster=w65, "Core.Current VI Reference"=w60, "Core.Close Panel on Exit?"=w64, "Synchronize.Echo.VIRef"=w60) -> (w70:T7)
        n30 = call <vilib>:"Add State(s) to Queue__JKI_lib_State_Machine.vi"("State(s) in (\"\")"=w72) -> ("States Out"=w71:string)  [unwired: 14 in]
      }
      frame "Error Handler" {
        # "Handle any errors here.\nYou can also output any states to clean-up after errors occur"
        # "Clear error"
        n31 = call <vilib>:"Add State(s) to Queue__JKI_lib_State_Machine.vi"("State(s) in Front (\"\")"="/* Post Error States", "State(s) in (\"\")"=w77) -> ("States Out"=w76:string)  [unwired: 13 in]
      }
      frame "Exit" {
        # "Do not put any code in this frame.\n(No errors that occur here will be handled.)"
        n32 = call <vilib>:"Add State(s) to Queue__JKI_lib_State_Machine.vi"("State(s) in (\"\")"=w82) -> ("States Out"=w81:string)  [unwired: 14 in]
      }
      frame "---------- Data ----------" {
        # "Do not put any code in this frame.\n(It is a separator no-op. You can make a copy of this frame to create a new Data frame)"
        n33 = call <vilib>:"Add State(s) to Queue__JKI_lib_State_Machine.vi"("State(s) in (\"\")"=w86) -> ("States Out"=w85:string)  [unwired: 14 in]
      }
      frame "Data: Initialize" {
        w88 = cluster{"VariableRef":T3} {"VariableRef"=refnum}  # Parameter
        w90 = T8 {"EnqueueData"={"Action"=enum."Create", "Data"=variant}, "Echo"={"VIRef"=refnum, "JsonOut"="", "Status"=""}, "Communicate"={"ID"="", "JsonIn"="", "VarRef"=refnum}, "Queue"=refnum}  # Synchronize
        w91 = T9 {"Current VI Reference"=refnum, "Close Panel on Exit?"=FALSE}  # Core
        n34 = Bundle("Core"=w91, "Parameter"=w88, "Synchronize"=w90, "FileClusters"=w87) -> (w89:T7)  [unwired: 1 in]
        n35 = call <vilib>:"Add State(s) to Queue__JKI_lib_State_Machine.vi"("State(s) in (\"\")"=w94) -> ("States Out"=w93:string)  [unwired: 14 in]
      }
      frame "Data: Cleanup" {
        # "Cleanup any data and references, here.\n(this is called automatically, by the Macro: Exit)"
        n36 = Unbundle By Name(w95) -> ("Core.Current VI Reference"=w98:refnum<vi>)
        n37 = Close Reference(reference=w98, error in (no error)=w97) -> (error out=w96:errorcluster)
        n38 = call <vilib>:"Add State(s) to Queue__JKI_lib_State_Machine.vi"("State(s) in (\"\")"=w100) -> ("States Out"=w99:string)  [unwired: 14 in]
      }
      frame "---------- UI ----------" {
        # "Do not put any code in this frame.\n(It is a separator no-op. You can make a copy of this frame to create a new UI frame)"
        n39 = call <vilib>:"Add State(s) to Queue__JKI_lib_State_Machine.vi"("State(s) in (\"\")"=w104) -> ("States Out"=w103:string)  [unwired: 14 in]
      }
      frame "UI: Initialize" {
        n40 = local write "Tab Control"(enum32{"Config", "控件"}."Config" ("Tab Control")) -> ()
        n41 = call <vilib>:"Add State(s) to Queue__JKI_lib_State_Machine.vi"("State(s) in (\"\")"=w109) -> ("States Out"=w108:string)  [unwired: 14 in]
      }
      frame "UI: Cursor Set" {
        # "Argument"
        # "Set and Unset Cursor Busy.\n(Usage: \"UI: Cursor Set >> Busy|Idle\")"
        n42 = case shown="\"Idle\", Default" w110 {
          tunnel: w112 -> [w117 w119]
          tunnel: [w116 w118] -> w111
          frame "Idle", Default {
            n43 = call <vilib>:"Unset Busy.vi"("error in (no error)"=w117) -> ("error out"=w116:errorcluster)  [unwired: 10 in]
          }
          frame "Busy" {
            n44 = call <vilib>:"Set Busy.vi"("error in (no error)"=w119) -> ("error out"=w118:errorcluster)  [unwired: 9 in, 1 out]
          }
        }
        n45 = call <vilib>:"Add State(s) to Queue__JKI_lib_State_Machine.vi"("State(s) in (\"\")"=w115) -> ("States Out"=w114:string)  [unwired: 14 in]
      }
      frame "UI: Initialize VarList" {
        n46 = call "GetVariables.vi"("error in (no error)"=w123, "VariableType"=enum16{"String", "StringArray"}."String", "DicRef"="VariablesRef") -> ("error out"=w122:errorcluster, "VariableArray"=w121:string[])  [unwired: 7 in]
        n47 = for {
          tunnel: w121 -> [w129] mode=indexing
          tunnel: [w130] -> w120 mode=indexing
          n48 = Bundle By Name(cluster=cluster{"String":string, "Value":string} {"String"="", "Value"=""}, "String"=w129, "Value"=w129) -> (w130:cluster{"String":string, "Value":string})
        }
        n49 = property on="路径(Path)" class="CmbBox"("Strings And Values[]"=w120) -> ()  [unwired: 2 in, 2 out]
        n50 = property on="二进制_WriteBinFile" class="CmbBox"("Strings And Values[]"=w120) -> ()  [unwired: 2 in, 2 out]
        n51 = property on="文本_WriteTextFile" class="CmbBox"("Strings And Values[]"=w120) -> ()  [unwired: 2 in, 2 out]
        n52 = call <vilib>:"Add State(s) to Queue__JKI_lib_State_Machine.vi"("State(s) in (\"\")"=w128) -> ("States Out"=w127:string)  [unwired: 14 in]
      }
      frame "UI: Front Panel State" {
        # "Argument"
        n53 = Unbundle By Name(w134) -> ("Core.Current VI Reference"=w133:refnum<vi>)
        n54 = case shown="\"Open\", \"Standard\", Default" w132 {
          tunnel: w136 -> [w144 w159 w170 w183 w196]
          tunnel: [w146 w160 w172 w185 w198] -> w135
          tunnel: w133 -> [w145 w157 w171 w184 w197]
          frame "Open", "Standard", Default {
            w139 = T5."Standard" ("State")
            n55 = property class="VI"(reference=w145, error in=w144) -> (reference out=w142:refnum<vi>, error out=w143:errorcluster, "FP.State"=w141:T5)
            n56 = Not Equal?(x=w141, y=w139) -> (x != y?=w140:bool)
            n57 = case shown="True" w140 {
              tunnel: [w150 w152] -> w146
              tunnel: w143 -> [w149 w152]
              tunnel: w142 -> [w148 _]
              tunnel: w139 -> [w147 _]
              frame True {
                n58 = invoke class="VI" method="FP.Open"(reference=w148, error in=w149, "Activate"=TRUE, "State"=w147) -> (error out=w150:errorcluster)  [unwired: 1 in, 4 out]
              }
              frame False {
              }
            }
          }
          frame "Close", "Closed" {
            n59 = property class="VI"(reference=w157, error in=w159) -> (reference out=w156:refnum<vi>, error out=w158:errorcluster, "FP.State"=w154:T5)
            n60 = Not Equal?(x=w154, y=T5."Closed" ("Front Panel Window:State")) -> (x != y?=w153:bool)
            n61 = case shown="True" w153 {
              tunnel: [w161 w164] -> w160
              tunnel: w158 -> [w161 w163]
              tunnel: w156 -> [_ w162]
              frame False {
              }
              frame True {
                n62 = invoke class="VI" method="FP.Close"(reference=w162, error in=w163) -> (error out=w164:errorcluster)  [unwired: 1 in, 2 out]
              }
            }
          }
          frame "Hidden", "Hide" {
            w165 = T5."Hidden" ("State")
            n63 = property class="VI"(reference=w171, error in=w170) -> (reference out=w168:refnum<vi>, error out=w169:errorcluster, "FP.State"=w167:T5)
            n64 = Not Equal?(x=w167, y=w165) -> (x != y?=w166:bool)
            n65 = case shown="True" w166 {
              tunnel: [w176 w177] -> w172
              tunnel: w169 -> [w175 w177]
              tunnel: w168 -> [w174 _]
              tunnel: w165 -> [w173 _]
              frame True {
                n66 = invoke class="VI" method="FP.Open"(reference=w174, error in=w175, "State"=w173) -> (error out=w176:errorcluster)  [unwired: 2 in, 4 out]
              }
              frame False {
              }
            }
          }
          frame "Minimize", "Minimized" {
            w178 = T5."Minimized" ("State")
            n67 = property class="VI"(reference=w184, error in=w183) -> (reference out=w181:refnum<vi>, error out=w182:errorcluster, "FP.State"=w180:T5)
            n68 = Not Equal?(x=w180, y=w178) -> (x != y?=w179:bool)
            n69 = case shown="True" w179 {
              tunnel: [w189 w190] -> w185
              tunnel: w182 -> [w188 w190]
              tunnel: w181 -> [w187 _]
              tunnel: w178 -> [w186 _]
              frame True {
                n70 = invoke class="VI" method="FP.Open"(reference=w187, error in=w188, "State"=w186) -> (error out=w189:errorcluster)  [unwired: 2 in, 4 out]
              }
              frame False {
              }
            }
          }
          frame "Maximize", "Maximized" {
            w191 = T5."Maximized" ("State")
            n71 = property class="VI"(reference=w197, error in=w196) -> (reference out=w194:refnum<vi>, error out=w195:errorcluster, "FP.State"=w193:T5)
            n72 = Not Equal?(x=w193, y=w191) -> (x != y?=w192:bool)
            n73 = case shown="True" w192 {
              tunnel: [w202 w203] -> w198
              tunnel: w195 -> [w201 w203]
              tunnel: w194 -> [w200 _]
              tunnel: w191 -> [w199 _]
              frame True {
                n74 = invoke class="VI" method="FP.Open"(reference=w200, error in=w201, "State"=w199) -> (error out=w202:errorcluster)  [unwired: 2 in, 4 out]
              }
              frame False {
              }
            }
          }
        }
        n75 = call <vilib>:"Add State(s) to Queue__JKI_lib_State_Machine.vi"("State(s) in (\"\")"=w138) -> ("States Out"=w137:string)  [unwired: 14 in]
      }
      frame "---------- Macro ----------" {
        n76 = call <vilib>:"Add State(s) to Queue__JKI_lib_State_Machine.vi"("State(s) in (\"\")"=w207) -> ("States Out"=w206:string)  [unwired: 14 in]
      }
      frame "Macro: Initialize" {
        n77 = call <vilib>:"Add State(s) to Queue__JKI_lib_State_Machine.vi"("State(s) in Front (\"\")"="Data: Initialize\nInitialize Core Data\nUI: Initialize\nSync: Obtain CMD Queue\nSync: Dequeue CMD\nUI: Initialize VarList\nParameter: Parse Parameter", "State(s) in (\"\")"=w212) -> ("States Out"=w211:string)  [unwired: 13 in]
      }
      frame "Macro: Exit" {
        n78 = Unbundle By Name(w219) -> ("Core.Close Panel on Exit?"=w218:bool)
        n79 = Select(t="UI: Front Panel State >> Close", s=w218, f="") -> (s? t:f=w215:string)
        n80 = call <vilib>:"Add State(s) to Queue__JKI_lib_State_Machine.vi"("State(s) in (\"\")"=w215, "State(s) at Back (\"\")"="Sync: Release CMD Queue\nData: Cleanup\nExit") -> ("States Out"=w213:string)  [unwired: 13 in]
        n81 = call <vilib>:"Add State(s) to Queue__JKI_lib_State_Machine.vi"("State(s) in Front (\"\")"=w213, "State(s) in (\"\")"=w222) -> ("States Out"=w221:string)  [unwired: 13 in]
      }
      frame "---------- Parameter ----------" {
        # "Template Separator\n(You can make a copy of, or modify, this frame)"
        n82 = call <vilib>:"Add State(s) to Queue__JKI_lib_State_Machine.vi"("State(s) in (\"\")"=w226) -> ("States Out"=w225:string)  [unwired: 14 in]
      }
      frame "Parameter: Parse Parameter" {
        n83 = Unbundle By Name(w229) -> ("FileClusters"=w228:T4)
        n84 = Empty String/Path?(string/path="In") -> (empty?=w232:bool)
        n85 = case shown="False" w232 {
          tunnel: "In" -> [w243 _]
          tunnel: w231 -> [w248 w445]
          tunnel: [w247 w445] -> w230
          tunnel: w228 -> [w246 _]
          frame False {
            n86 = Match Pattern(string=w243, regular expression="\"Method\":\"") -> (after substring=w242:string)  [unwired: 1 in, 3 out]
            n87 = Match Pattern(string=w242, regular expression="\",") -> (before substring=w241:string)  [unwired: 1 in, 3 out]
            n88 = case shown="\"WriteBinFile\"" w241 {
              tunnel: w243 -> [w262 w285 w295 w307 w318 w336 w353 w371 w381 w393 w405 w415 w425 w441 _]
              tunnel: w248 -> [w260 w283 w293 w305 w316 w334 w351 w369 w379 w391 w403 w413 w423 w439 w444]
              tunnel: [w259 w282 w292 w304 w315 w333 w350 w368 w378 w390 w402 w412 w422 w438 w444] -> w247
              tunnel: w246 -> [w257 w280 w290 w302 w313 w331 w348 w366 w376 w388 w400 w410 w420 w436 _]
              tunnel: [w258 w281 w291 w303 w314 w332 w349 w367 w377 w389 w401 w411 w421 w437 _] -> w236
              frame "SetPath" {
                n89 = Unbundle By Name(w257) -> ("SetPath"=w256:T10)
                n90 = call <vilib>:"Unflatten From JSON String.vi"("Type and Defaults"=w256, "error in (no error)"=w260, "JSON String"=w262) -> ("error out"=w263:errorcluster, "Variant"=w264:variant)  [unwired: 7 in]
                n91 = Variant To Data(error in=w263, type=w256, Variant=w264) -> (data=w261:T10, error out=w259:errorcluster)
                n92 = Unbundle By Name(w261) -> ("json.Method"=w258:string, "json.Path"=w255:string, "json.PathType"=w250:string)
                n93 = local write "路径(Path)"(w255) -> ()
                n94 = property on="路径类型_SetPath" class="Ring (strict)"() -> ("Strings []"=w251:string[])  [unwired: 2 in, 2 out]
                n95 = Search 1D Array(1D array=w251, element=w250) -> (index of element=w254:i32)  [unwired: 1 in]
                n96 = Greater Or Equal To 0?(x=w254) -> (x >= 0?=w253:bool)
                n97 = Select(t=w254, s=w253, f=0) -> (s? t:f=w249:i32)
                n98 = property on="路径类型_SetPath" class="Ring (strict)"("Value"=w249) -> ()  [unwired: 2 in, 2 out]
              }
              frame "CreatFile" {
                n99 = Unbundle By Name(w280) -> ("CreatFile"=w279:T11)
                n100 = call <vilib>:"Unflatten From JSON String.vi"("Type and Defaults"=w279, "error in (no error)"=w283, "JSON String"=w285) -> ("error out"=w286:errorcluster, "Variant"=w287:variant)  [unwired: 7 in]
                n101 = Variant To Data(error in=w286, type=w279, Variant=w287) -> (data=w284:T11, error out=w282:errorcluster)
                n102 = Unbundle By Name(w284) -> ("json.Method"=w281:string, "json.Path"=w278:string, "json.Operation"=w274:string, "json.Access"=w270:string, "json.DisableBuffering"=w265:bool)
                n103 = local write "禁用缓存_CreatFile"(w265) -> ()
                n104 = property on="操作_CreatFile" class="Ring (strict)"() -> ("Strings []"=w269:string[])  [unwired: 2 in, 2 out]
                n105 = property on="权限_CreatFile" class="Ring (strict)"() -> ("Strings []"=w267:string[])  [unwired: 2 in, 2 out]
                n106 = local write "路径(Path)"(w278) -> ()
                n107 = Search 1D Array(1D array=w269, element=w274) -> (index of element=w277:i32)  [unwired: 1 in]
                n108 = Search 1D Array(1D array=w267, element=w270) -> (index of element=w273:i32)  [unwired: 1 in]
                n109 = Greater Or Equal To 0?(x=w277) -> (x >= 0?=w276:bool)
                n110 = Greater Or Equal To 0?(x=w273) -> (x >= 0?=w272:bool)
                n111 = Select(t=w277, s=w276, f=0) -> (s? t:f=w268:i32)
                n112 = Select(t=w273, s=w272, f=0) -> (s? t:f=w266:i32)
                n113 = property on="权限_CreatFile" class="Ring (strict)"("Value"=w266) -> ()  [unwired: 2 in, 2 out]
                n114 = property on="操作_CreatFile" class="Ring (strict)"("Value"=w268) -> ()  [unwired: 2 in, 2 out]
              }
              frame "CreatFolder" {
                n115 = Unbundle By Name(w290) -> ("CreatFolder"=w289:T12)
                n116 = call <vilib>:"Unflatten From JSON String.vi"("Type and Defaults"=w289, "error in (no error)"=w293, "JSON String"=w295) -> ("error out"=w296:errorcluster, "Variant"=w297:variant)  [unwired: 7 in]
                n117 = Variant To Data(error in=w296, type=w289, Variant=w297) -> (data=w294:T12, error out=w292:errorcluster)
                n118 = Unbundle By Name(w294) -> ("json.Method"=w291:string, "json.Path"=w288:string)
                n119 = local write "路径(Path)"(w288) -> ()
              }
              frame "Delete" {
                n120 = Unbundle By Name(w302) -> ("Delete"=w301:T13)
                n121 = call <vilib>:"Unflatten From JSON String.vi"("Type and Defaults"=w301, "error in (no error)"=w305, "JSON String"=w307) -> ("error out"=w308:errorcluster, "Variant"=w309:variant)  [unwired: 7 in]
                n122 = Variant To Data(error in=w308, type=w301, Variant=w309) -> (data=w306:T13, error out=w304:errorcluster)
                n123 = Unbundle By Name(w306) -> ("json.Method"=w303:string, "json.Path"=w300:string, "json.EntireHierarchy"=w299:bool, "json.Confirm"=w298:bool)
                n124 = local write "完整层次结构_Delete"(w299) -> ()
                n125 = local write "手动确认_Delete"(w298) -> ()
                n126 = local write "路径(Path)"(w300) -> ()
              }
              frame "ReadTextFile" {
                n127 = Unbundle By Name(w313) -> ("ReadTextFile"=w312:T14)
                n128 = call <vilib>:"Unflatten From JSON String.vi"("Type and Defaults"=w312, "error in (no error)"=w316, "JSON String"=w318) -> ("error out"=w319:errorcluster, "Variant"=w320:variant)  [unwired: 7 in]
                n129 = Variant To Data(error in=w319, type=w312, Variant=w320) -> (data=w317:T14, error out=w315:errorcluster)
                n130 = Unbundle By Name(w317) -> ("json.Method"=w314:string, "json.Path"=w311:string, "json.count"=w310:i32)
                n131 = local write "计数_ReadTextFile"(w310) -> ()
                n132 = local write "路径(Path)"(w311) -> ()
              }
              frame "WriteTextFile" {
                n133 = Unbundle By Name(w331) -> ("WriteTextFile"=w330:T15)
                n134 = call <vilib>:"Unflatten From JSON String.vi"("Type and Defaults"=w330, "error in (no error)"=w334, "JSON String"=w336) -> ("error out"=w337:errorcluster, "Variant"=w338:variant)  [unwired: 7 in]
                n135 = Variant To Data(error in=w337, type=w330, Variant=w338) -> (data=w335:T15, error out=w333:errorcluster)
                n136 = Unbundle By Name(w335) -> ("json.Method"=w332:string, "json.Path"=w329:string, "json.Offset"=w328:i64, "json.Position"=w323:string, "json.Text"=w321:string)
                n137 = property on="起始位置_WriteTextFile" class="Ring (strict)"() -> ("Strings []"=w324:string[])  [unwired: 2 in, 2 out]
                n138 = local write "文本_WriteTextFile"(w321) -> ()
                n139 = local write "偏移_WriteTextFile"(w328) -> ()
                n140 = Search 1D Array(1D array=w324, element=w323) -> (index of element=w327:i32)  [unwired: 1 in]
                n141 = Greater Or Equal To 0?(x=w327) -> (x >= 0?=w326:bool)
                n142 = local write "路径(Path)"(w329) -> ()
                n143 = Select(t=w327, s=w326, f=0) -> (s? t:f=w322:i32)
                n144 = property on="起始位置_WriteTextFile" class="Ring (strict)"("Value"=w322) -> ()  [unwired: 2 in, 2 out]
              }
              frame "ReadBinFile" {
                n145 = Unbundle By Name(w348) -> ("ReadBinFile"=w347:T16)
                n146 = call <vilib>:"Unflatten From JSON String.vi"("Type and Defaults"=w347, "error in (no error)"=w351, "JSON String"=w353) -> ("error out"=w354:errorcluster, "Variant"=w355:variant)  [unwired: 7 in]
                n147 = Variant To Data(error in=w354, type=w347, Variant=w355) -> (data=w352:T16, error out=w350:errorcluster)
                n148 = Unbundle By Name(w352) -> ("json.Method"=w349:string, "json.Path"=w346:string, "json.Count"=w341:i32, "json.ByteOrder"=w342:string)
                n149 = property on="字节顺序_ReadBinFile" class="Ring (strict)"() -> ("Strings []"=w340:string[])  [unwired: 2 in, 2 out]
                n150 = local write "计数_ReadBinFile"(w341) -> ()
                n151 = Search 1D Array(1D array=w340, element=w342) -> (index of element=w345:i32)  [unwired: 1 in]
                n152 = local write "路径(Path)"(w346) -> ()
                n153 = Greater Or Equal To 0?(x=w345) -> (x >= 0?=w344:bool)
                n154 = Select(t=w345, s=w344, f=0) -> (s? t:f=w339:i32)
                n155 = property on="字节顺序_ReadBinFile" class="Ring (strict)"("Value"=w339) -> ()  [unwired: 2 in, 2 out]
              }
              frame "WriteBinFile" {
                n156 = Unbundle By Name(w366) -> ("WriteBinFile"=w365:T17)
                n157 = call <vilib>:"Unflatten From JSON String.vi"("Type and Defaults"=w365, "error in (no error)"=w369, "JSON String"=w371) -> ("error out"=w372:errorcluster, "Variant"=w373:variant)  [unwired: 7 in]
                n158 = Variant To Data(error in=w372, type=w365, Variant=w373) -> (data=w370:T17, error out=w368:errorcluster)
                n159 = Unbundle By Name(w370) -> ("json.Method"=w367:string, "json.Path"=w364:string, "json.ByteOrder"=w360:string, "json.PrependDataSize"=w359:bool, "json.Bin"=w356:string)
                n160 = local write "二进制_WriteBinFile"(w356) -> ()
                n161 = local write "前置数据大小_WriteBinFile"(w359) -> ()
                n162 = property on="字节顺序_WriteBinFile" class="Ring (strict)"() -> ("Strings []"=w358:string[])  [unwired: 2 in, 2 out]
                n163 = local write "路径(Path)"(w364) -> ()
                n164 = Search 1D Array(1D array=w358, element=w360) -> (index of element=w363:i32)  [unwired: 1 in]
                n165 = Greater Or Equal To 0?(x=w363) -> (x >= 0?=w362:bool)
                n166 = Select(t=w363, s=w362, f=0) -> (s? t:f=w357:i32)
                n167 = property on="字节顺序_WriteBinFile" class="Ring (strict)"("Value"=w357) -> ()  [unwired: 2 in, 2 out]
              }
              frame "ReadFileMD5" {
                n168 = Unbundle By Name(w376) -> ("ReadFileMD5"=w375:T12)
                n169 = call <vilib>:"Unflatten From JSON String.vi"("Type and Defaults"=w375, "error in (no error)"=w379, "JSON String"=w381) -> ("error out"=w382:errorcluster, "Variant"=w383:variant)  [unwired: 7 in]
                n170 = Variant To Data(error in=w382, type=w375, Variant=w383) -> (data=w380:T12, error out=w378:errorcluster)
                n171 = Unbundle By Name(w380) -> ("json.Method"=w377:string, "json.Path"=w374:string)
                n172 = local write "路径(Path)"(w374) -> ()
              }
              frame "Move" {
                n173 = Unbundle By Name(w388) -> ("Move"=w387:T18)
                n174 = call <vilib>:"Unflatten From JSON String.vi"("Type and Defaults"=w387, "error in (no error)"=w391, "JSON String"=w393) -> ("error out"=w394:errorcluster, "Variant"=w395:variant)  [unwired: 7 in]
                n175 = Variant To Data(error in=w394, type=w387, Variant=w395) -> (data=w392:T18, error out=w390:errorcluster)
                n176 = Unbundle By Name(w392) -> ("json.Method"=w389:string, "json.Path"=w386:string, "json.TargetPath"=w385:string, "json.Overwrite"=w384:bool)
                n177 = local write "覆盖_Move"(w384) -> ()
                n178 = local write "文件路径_Move"(w385) -> ()
                n179 = local write "路径(Path)"(w386) -> ()
              }
              frame "Copy" {
                n180 = Unbundle By Name(w400) -> ("Copy"=w399:T18)
                n181 = call <vilib>:"Unflatten From JSON String.vi"("Type and Defaults"=w399, "error in (no error)"=w403, "JSON String"=w405) -> ("error out"=w406:errorcluster, "Variant"=w407:variant)  [unwired: 7 in]
                n182 = Variant To Data(error in=w406, type=w399, Variant=w407) -> (data=w404:T18, error out=w402:errorcluster)
                n183 = Unbundle By Name(w404) -> ("json.Method"=w401:string, "json.Path"=w398:string, "json.TargetPath"=w397:string, "json.Overwrite"=w396:bool)
                n184 = local write "目标文件路径_Copy"(w397) -> ()
                n185 = local write "覆盖_Copy"(w396) -> ()
                n186 = local write "路径(Path)"(w398) -> ()
              }
              frame "GetFileSize" {
                n187 = Unbundle By Name(w410) -> ("GetFileSize"=w409:T12)
                n188 = call <vilib>:"Unflatten From JSON String.vi"("Type and Defaults"=w409, "error in (no error)"=w413, "JSON String"=w415) -> ("error out"=w416:errorcluster, "Variant"=w417:variant)  [unwired: 7 in]
                n189 = Variant To Data(error in=w416, type=w409, Variant=w417) -> (data=w414:T12, error out=w412:errorcluster)
                n190 = Unbundle By Name(w414) -> ("json.Method"=w411:string, "json.Path"=w408:string)
                n191 = local write "路径(Path)"(w408) -> ()
              }
              frame "CheckifFileorFolderExists" {
                n192 = Unbundle By Name(w420) -> ("CheckifFileorFolderExists"=w419:T12)
                n193 = call <vilib>:"Unflatten From JSON String.vi"("Type and Defaults"=w419, "error in (no error)"=w423, "JSON String"=w425) -> ("error out"=w426:errorcluster, "Variant"=w427:variant)  [unwired: 7 in]
                n194 = Variant To Data(error in=w426, type=w419, Variant=w427) -> (data=w424:T12, error out=w422:errorcluster)
                n195 = Unbundle By Name(w424) -> ("json.Method"=w421:string, "json.Path"=w418:string)
                n196 = local write "路径(Path)"(w418) -> ()
              }
              frame "ListFolder" {
                n197 = Unbundle By Name(w436) -> ("ListFolder"=w435:T19)
                n198 = call <vilib>:"Unflatten From JSON String.vi"("Type and Defaults"=w435, "error in (no error)"=w439, "JSON String"=w441) -> ("error out"=w442:errorcluster, "Variant"=w443:variant)  [unwired: 7 in]
                n199 = Variant To Data(error in=w442, type=w435, Variant=w443) -> (data=w440:T19, error out=w438:errorcluster)
                n200 = Unbundle By Name(w440) -> ("json.Method"=w437:string, "json.Path"=w434:string, "json.Type"=w429:string)
                n201 = property on="类型_ListFolder" class="Ring (strict)"() -> ("Strings []"=w430:string[])  [unwired: 2 in, 2 out]
                n202 = Search 1D Array(1D array=w430, element=w429) -> (index of element=w433:i32)  [unwired: 1 in]
                n203 = Greater Or Equal To 0?(x=w433) -> (x >= 0?=w432:bool)
                n204 = Select(t=w433, s=w432, f=0) -> (s? t:f=w428:i32)
                n205 = local write "路径(Path)"(w434) -> ()
                n206 = property on="类型_ListFolder" class="Ring (strict)"("Value"=w428) -> ()  [unwired: 2 in, 2 out]
              }
              frame Default {
              }
            }
            n207 = property on="方法(Method)" class="Enum (strict)"() -> ("Strings []"=w238:string[])  [unwired: 2 in, 2 out]
            n208 = Search 1D Array(1D array=w238, element=w236) -> (index of element=w240:i32)  [unwired: 1 in]
            n209 = Greater Or Equal To 0?(x=w240) -> (x >= 0?=w239:bool)
            n210 = Select(t=w240, s=w239, f=0) -> (s? t:f=w235:i32)
            n211 = local write "Type"(w235) -> ()
            n212 = property on="方法(Method)" class="Enum (strict)"("Value"=w235) -> ()  [unwired: 2 in, 2 out]
          }
          frame True {
          }
        }
        n213 = call <vilib>:"Add State(s) to Queue__JKI_lib_State_Machine.vi"("State(s) in (\"\")"=w234) -> ("States Out"=w233:string)  [unwired: 14 in]
      }
      frame "Parameter: Combin Parameter" {
        n214 = Unbundle By Name(w447) -> ("FileClusters"=w446:T4)
        n215 = property on="方法(Method)" class="Enum (strict)"() -> ("RingText.Text"=w449:string)  [unwired: 2 in, 2 out]
        n216 = case shown="\"WriteBinFile\"" w449 {
          selector: w449 -> [_ w459 w471 w480 w491 w501 w513 w524 w536 w545 w556 w567 w576 w585 w595]
          tunnel: w446 -> [_ w465 w477 w486 w497 w507 w519 w530 w542 w551 w562 w573 w582 w591 w601]
          tunnel: [_ w463 w475 w484 w495 w505 w517 w528 w540 w549 w560 w571 w580 w589 w599] -> w448
          tunnel: [w455 w458 w470 w479 w490 w500 w512 w523 w535 w544 w555 w566 w575 w584 w594] -> w451
          tunnel: w450 -> [w455 w461 w473 w482 w493 w503 w515 w526 w538 w547 w558 w569 w578 w587 w597]
          frame Default {
          }
          frame "SetPath" {
            n217 = local read "路径(Path)"() -> (w457:string)
            n218 = property on="路径类型_SetPath" class="Ring (strict)"() -> ("RingText.Text"=w456:string)  [unwired: 2 in, 2 out]
            n219 = Unbundle By Name(w465) -> ("SetPath"=w464:T10)
            n220 = Bundle By Name(cluster=w464, "json.Method"=w459, "json.Path"=w457, "json.PathType"=w456) -> (w460:T10)
            n221 = call <vilib>:"Flatten To JSON String.vi"("Multiline (T)"=TRUE, "error in (no error)"=w461, "Variant"=w460) -> ("error out"=w458:errorcluster, "JSON String"=w463:string)  [unwired: 7 in]
          }
          frame "CreatFile" {
            n222 = local read "禁用缓存_CreatFile"() -> (w466:bool)
            n223 = property on="操作_CreatFile" class="Ring (strict)"() -> ("RingText.Text"=w468:string)  [unwired: 2 in, 2 out]
            n224 = property on="权限_CreatFile" class="Ring (strict)"() -> ("RingText.Text"=w467:string)  [unwired: 2 in, 2 out]
            n225 = local read "路径(Path)"() -> (w469:string)
            n226 = Unbundle By Name(w477) -> ("CreatFile"=w476:T11)
            n227 = Bundle By Name(cluster=w476, "json.Method"=w471, "json.Path"=w469, "json.Operation"=w468, "json.Access"=w467, "json.DisableBuffering"=w466) -> (w472:T11)
            n228 = call <vilib>:"Flatten To JSON String.vi"("Multiline (T)"=TRUE, "error in (no error)"=w473, "Variant"=w472) -> ("error out"=w470:errorcluster, "JSON String"=w475:string)  [unwired: 7 in]
          }
          frame "CreatFolder" {
            n229 = local read "路径(Path)"() -> (w478:string)
            n230 = Unbundle By Name(w486) -> ("CreatFolder"=w485:T12)
            n231 = Bundle By Name(cluster=w485, "json.Method"=w480, "json.Path"=w478) -> (w481:T12)
            n232 = call <vilib>:"Flatten To JSON String.vi"("Multiline (T)"=TRUE, "error in (no error)"=w482, "Variant"=w481) -> ("error out"=w479:errorcluster, "JSON String"=w484:string)  [unwired: 7 in]
          }
          frame "Delete" {
            n233 = local read "完整层次结构_Delete"() -> (w488:bool)
            n234 = local read "手动确认_Delete"() -> (w487:bool)
            n235 = local read "路径(Path)"() -> (w489:string)
            n236 = Unbundle By Name(w497) -> ("Delete"=w496:T13)
            n237 = Bundle By Name(cluster=w496, "json.Method"=w491, "json.Path"=w489, "json.EntireHierarchy"=w488, "json.Confirm"=w487) -> (w492:T13)
            n238 = call <vilib>:"Flatten To JSON String.vi"("Multiline (T)"=TRUE, "error in (no error)"=w493, "Variant"=w492) -> ("error out"=w490:errorcluster, "JSON String"=w495:string)  [unwired: 7 in]
          }
          frame "ReadTextFile" {
            n239 = local read "计数_ReadTextFile"() -> (w498:i32)
            n240 = local read "路径(Path)"() -> (w499:string)
            n241 = Unbundle By Name(w507) -> ("ReadTextFile"=w506:T14)
            n242 = Bundle By Name(cluster=w506, "json.Method"=w501, "json.Path"=w499, "json.count"=w498) -> (w502:T14)
            n243 = call <vilib>:"Flatten To JSON String.vi"("Multiline (T)"=TRUE, "error in (no error)"=w503, "Variant"=w502) -> ("error out"=w500:errorcluster, "JSON String"=w505:string)  [unwired: 7 in]
          }
          frame "WriteTextFile" {
            n244 = local read "偏移_WriteTextFile"() -> (w510:i64)
            n245 = property on="起始位置_WriteTextFile" class="Ring (strict)"() -> ("RingText.Text"=w509:string)  [unwired: 2 in, 2 out]
            n246 = local read "文本_WriteTextFile"() -> (w508:string)
            n247 = local read "路径(Path)"() -> (w511:string)
            n248 = Unbundle By Name(w519) -> ("WriteTextFile"=w518:T15)
            n249 = Bundle By Name(cluster=w518, "json.Method"=w513, "json.Path"=w511, "json.Offset"=w510, "json.Position"=w509, "json.Text"=w508) -> (w514:T15)
            n250 = call <vilib>:"Flatten To JSON String.vi"("Multiline (T)"=TRUE, "error in (no error)"=w515, "Variant"=w514) -> ("error out"=w512:errorcluster, "JSON String"=w517:string)  [unwired: 7 in]
          }
          frame "ReadBinFile" {
            n251 = local read "计数_ReadBinFile"() -> (w521:i32)
            n252 = property on="字节顺序_ReadBinFile" class="Ring (strict)"() -> ("RingText.Text"=w520:string)  [unwired: 2 in, 2 out]
            n253 = local read "路径(Path)"() -> (w522:string)
            n254 = Unbundle By Name(w530) -> ("ReadBinFile"=w529:T16)
            n255 = Bundle By Name(cluster=w529, "json.Method"=w524, "json.Path"=w522, "json.Count"=w521, "json.ByteOrder"=w520) -> (w525:T16)
            n256 = call <vilib>:"Flatten To JSON String.vi"("Multiline (T)"=TRUE, "error in (no error)"=w526, "Variant"=w525) -> ("error out"=w523:errorcluster, "JSON String"=w528:string)  [unwired: 7 in]
          }
          frame "WriteBinFile" {
            n257 = local read "前置数据大小_WriteBinFile"() -> (w532:bool)
            n258 = property on="字节顺序_WriteBinFile" class="Ring (strict)"() -> ("RingText.Text"=w533:string)  [unwired: 2 in, 2 out]
            n259 = local read "二进制_WriteBinFile"() -> (w531:string)
            n260 = local read "路径(Path)"() -> (w534:string)
            n261 = Unbundle By Name(w542) -> ("WriteBinFile"=w541:T17)
            n262 = Bundle By Name(cluster=w541, "json.Method"=w536, "json.Path"=w534, "json.ByteOrder"=w533, "json.PrependDataSize"=w532, "json.Bin"=w531) -> (w537:T17)
            n263 = call <vilib>:"Flatten To JSON String.vi"("Multiline (T)"=TRUE, "error in (no error)"=w538, "Variant"=w537) -> ("error out"=w535:errorcluster, "JSON String"=w540:string)  [unwired: 7 in]
          }
          frame "ReadFileMD5" {
            n264 = local read "路径(Path)"() -> (w543:string)
            n265 = Unbundle By Name(w551) -> ("ReadFileMD5"=w550:T12)
            n266 = Bundle By Name(cluster=w550, "json.Method"=w545, "json.Path"=w543) -> (w546:T12)
            n267 = call <vilib>:"Flatten To JSON String.vi"("Multiline (T)"=TRUE, "error in (no error)"=w547, "Variant"=w546) -> ("error out"=w544:errorcluster, "JSON String"=w549:string)  [unwired: 7 in]
          }
          frame "Move" {
            n268 = local read "文件路径_Move"() -> (w553:string)
            n269 = local read "覆盖_Move"() -> (w552:bool)
            n270 = local read "路径(Path)"() -> (w554:string)
            n271 = Unbundle By Name(w562) -> ("Move"=w561:T18)
            n272 = Bundle By Name(cluster=w561, "json.Method"=w556, "json.Path"=w554, "json.TargetPath"=w553, "json.Overwrite"=w552) -> (w557:T18)
            n273 = call <vilib>:"Flatten To JSON String.vi"("Multiline (T)"=TRUE, "error in (no error)"=w558, "Variant"=w557) -> ("error out"=w555:errorcluster, "JSON String"=w560:string)  [unwired: 7 in]
          }
          frame "Copy" {
            n274 = local read "目标文件路径_Copy"() -> (w564:string)
            n275 = local read "覆盖_Copy"() -> (w563:bool)
            n276 = local read "路径(Path)"() -> (w565:string)
            n277 = Unbundle By Name(w573) -> ("Copy"=w572:T18)
            n278 = Bundle By Name(cluster=w572, "json.Method"=w567, "json.Path"=w565, "json.TargetPath"=w564, "json.Overwrite"=w563) -> (w568:T18)
            n279 = call <vilib>:"Flatten To JSON String.vi"("Multiline (T)"=TRUE, "error in (no error)"=w569, "Variant"=w568) -> ("error out"=w566:errorcluster, "JSON String"=w571:string)  [unwired: 7 in]
          }
          frame "GetFileSize" {
            n280 = local read "路径(Path)"() -> (w574:string)
            n281 = Unbundle By Name(w582) -> ("GetFileSize"=w581:T12)
            n282 = Bundle By Name(cluster=w581, "json.Method"=w576, "json.Path"=w574) -> (w577:T12)
            n283 = call <vilib>:"Flatten To JSON String.vi"("Multiline (T)"=TRUE, "error in (no error)"=w578, "Variant"=w577) -> ("error out"=w575:errorcluster, "JSON String"=w580:string)  [unwired: 7 in]
          }
          frame "CheckifFileorFolderExists" {
            n284 = local read "路径(Path)"() -> (w583:string)
            n285 = Unbundle By Name(w591) -> ("CheckifFileorFolderExists"=w590:T12)
            n286 = Bundle By Name(cluster=w590, "json.Method"=w585, "json.Path"=w583) -> (w586:T12)
            n287 = call <vilib>:"Flatten To JSON String.vi"("Multiline (T)"=TRUE, "error in (no error)"=w587, "Variant"=w586) -> ("error out"=w584:errorcluster, "JSON String"=w589:string)  [unwired: 7 in]
          }
          frame "ListFolder" {
            n288 = property on="类型_ListFolder" class="Ring (strict)"() -> ("RingText.Text"=w592:string)  [unwired: 2 in, 2 out]
            n289 = local read "路径(Path)"() -> (w593:string)
            n290 = Unbundle By Name(w601) -> ("ListFolder"=w600:T19)
            n291 = Bundle By Name(cluster=w600, "json.Method"=w595, "json.Path"=w593, "json.Type"=w592) -> (w596:T19)
            n292 = call <vilib>:"Flatten To JSON String.vi"("Multiline (T)"=TRUE, "error in (no error)"=w597, "Variant"=w596) -> ("error out"=w594:errorcluster, "JSON String"=w599:string)  [unwired: 7 in]
          }
        }
        n293 = Bundle By Name(cluster=w447, "Synchronize.Echo.JsonOut"=w448) -> (w452:T7)
        n294 = call <vilib>:"Add State(s) to Queue__JKI_lib_State_Machine.vi"("State(s) in (\"\")"=w454) -> ("States Out"=w453:string)  [unwired: 14 in]
      }
      frame "---------- Sync ----------" {
        n295 = call <vilib>:"Add State(s) to Queue__JKI_lib_State_Machine.vi"("State(s) in (\"\")"=w605) -> ("States Out"=w604:string)  [unwired: 14 in]
      }
      frame "Sync: Obtain CMD Queue" {
        # "这里由平台输入"
        n296 = Unbundle By Name(w607) -> ("Synchronize.EnqueueData"=w606:T20)
        n297 = Obtain Queue(name (unnamed)="VIId", element data type=w606, error in (no error)=w612) -> (queue out=w608:refnum<queue>, error out=w611:errorcluster)  [unwired: 2 in, 1 out]
        n298 = Bundle By Name(cluster=w607, "Synchronize.Queue"=w608) -> (w609:T7)
        n299 = call <vilib>:"Add State(s) to Queue__JKI_lib_State_Machine.vi"("State(s) in (\"\")"=w614) -> ("States Out"=w613:string)  [unwired: 14 in]
      }
      frame "Sync: Dequeue CMD" {
        n300 = Unbundle By Name(w627) -> ("Synchronize.Queue"=w624:refnum<queue>, "Synchronize.Communicate"=w615:T21)
        n301 = Dequeue Element(queue=w624, timeout in ms (-1)=10, error in (no error)=w625) -> (queue out=w623:refnum<queue>, element=w621:T20, timed out?=w622:bool, error out=w617:errorcluster)
        n302 = Bundle By Name(cluster=w627, "Synchronize.Queue"=w623, "Synchronize.EnqueueData"=w621) -> (w619:T7)
        n303 = case shown="False" w622 {
          tunnel: w621 -> [w638 _]
          tunnel: [w636 _] -> w620
          tunnel: w619 -> [w635 w667]
          tunnel: [w634 w667] -> w618
          tunnel: w617 -> [w632 w666]
          tunnel: [w631 w666] -> w616
          tunnel: w615 -> [w630 _]
          frame False {
            n304 = Unbundle By Name(w638) -> ("Action"=w637:T22, "Data"=w633:variant)
            n305 = case shown="\"Query\"" w637 {
              tunnel: ["Sync: Send ECHO" "UI: Initialize VarList\nSync: Send ECHO" _ "Sync: Send ECHO\nMacro: Exit" "Parameter: Combin Parameter\nSync: Send ECHO" "Parameter: Parse Parameter\nSync: Send ECHO"] -> w636
              tunnel: w635 -> [w641 w646 w650 w653 w658 w663]
              tunnel: [w640 w645 w650 w652 w657 w662] -> w634
              tunnel: w633 -> [_ _ _ _ _ _]
              tunnel: w632 -> [w642 w647 w649 w654 w659 w664]
              tunnel: [w642 w647 w649 w654 w659 w664] -> w631
              tunnel: w630 -> [_ _ _ _ _ _]
              frame "Create" {
                n306 = Bundle By Name(cluster=w641, "Synchronize.Echo.Status"="Create Success") -> (w640:T7)
              }
              frame "UpdateVariable" {
                n307 = Bundle By Name(cluster=w646, "Synchronize.Echo.Status"="UpdateVariable Success") -> (w645:T7)
              }
              frame Default {
              }
              frame "Close" {
                n308 = Bundle By Name(cluster=w653, "Synchronize.Echo.Status"="Close Success") -> (w652:T7)
              }
              frame "Query" {
                n309 = Bundle By Name(cluster=w658, "Synchronize.Echo.Status"="Query Success") -> (w657:T7)
              }
              frame "Revert" {
                n310 = Bundle By Name(cluster=w663, "Synchronize.Echo.Status"="Revert Success") -> (w662:T7)
              }
            }
          }
          frame True {
          }
        }
        n311 = call <vilib>:"Add State(s) to Queue__JKI_lib_State_Machine.vi"("State(s) in Front (\"\")"=w620, "State(s) in (\"\")"=w629) -> ("States Out"=w628:string)  [unwired: 13 in]
      }
      frame "Sync: Release CMD Queue" {
        n312 = Unbundle By Name(w670) -> ("Synchronize.Queue"=w671:refnum<queue>)
        n313 = Release Queue(queue=w671, error in (no error)=w669) -> (error out=w668:errorcluster)  [unwired: 1 in, 2 out]
        n314 = call <vilib>:"Add State(s) to Queue__JKI_lib_State_Machine.vi"("State(s) in (\"\")"=w673) -> ("States Out"=w672:string)  [unwired: 14 in]
      }
      frame "Sync: Send ECHO" {
        n315 = Unbundle By Name(w677) -> ("Synchronize.Communicate"=w674:T21, "Synchronize.EnqueueData.Data"=w686:variant, "Synchronize.Echo"=w678:T23)
        n316 = Variant To Data(error in=w676, type=w674, Variant=w686) -> (data=w679:T21, error out=w680:errorcluster)
        n317 = Unbundle By Name(w679) -> ("ID"=w683:string)
        n318 = Obtain Queue(name (unnamed)=w683, element data type=w678, error in (no error)=w680) -> (queue out=w682:refnum<queue>, error out=w684:errorcluster)  [unwired: 2 in, 1 out]
        n319 = Enqueue Element(queue=w682, element=w678, error in (no error)=w684) -> (queue out=w681:refnum<queue>, error out=w685:errorcluster)  [unwired: 1 in, 1 out]
        n320 = Release Queue(queue=w681, error in (no error)=w685) -> (error out=w675:errorcluster)  [unwired: 1 in, 2 out]
        n321 = call <vilib>:"Add State(s) to Queue__JKI_lib_State_Machine.vi"("State(s) in (\"\")"=w688) -> ("States Out"=w687:string)  [unwired: 14 in]
      }
    }
  }
  n322 = flat-sequence {
    frame #0 {
    }
  }
